vi "Orca Flash Capture Manager.vi"(7 "Calling VI Ref":refnum<vi>) -> ()   [LabVIEW 2016]
uses:
  Orca Flash Capture Manager Controls/Orca Flash Capture Switch Line Scan Modes.ctl
  Orca Flash Capture Manager Controls/Orca Flash Capture Line Scan Settings.ctl
  Orca Flash Capture Manager Controls/Orca Flash Switch Cycles Steps.ctl
  <vilib>/Utility/miscctls.llb/LVPointTypeDef.ctl
  Orca Flash Capture Manager Controls/Orca Flash Capture Notifier Type.ctl
  Orca Flash Capture Manager Controls/Orca Flash Capture Actions.ctl
  <vilib>/vision/Image Controls.llb/IMAQ Image.ctl
  Hardware Configuration/Hardware Configuration Controls/Device Type.ctl
  Orca Flash Capture Manager Controls/Orca Flash Capture Line Scan Filter Settings.ctl
  Hardware Configuration/Hardware Configuration Controls/Device Function.ctl
  Device Library/Cameras/Hamamatsu/Orca Flash/Orca Flash Controls/Orca Flash Actions.ctl
  Device Library/Cameras/Hamamatsu/Orca Flash/Orca Flash Controls/Orca Flash Parameters.ctl
  Device Library/Cameras/Hamamatsu/Orca Flash/Orca Flash Controls/Orca Flash Parameter List.ctl
  Device Library/Cameras/Hamamatsu/Orca Flash/Orca Flash Controls/Orca Flash ROI.ctl
  Orca Flash Capture Manager Controls/Orca Flash Capture Cycle Step Count.ctl
  Device Manager/Common Device Queue/Common Device Controls/Common Device Actions.ctl
  Device Library/SMTP Email Alerts/SMTP Email Alerts Type Defs/SMTP Email Alerts Actions.ctl
  Device Library/DAQmx/AO Single Channel Triggered Ramp/AO SCTR Type Defs/AO SCTR Actions.ctl
  Wide Field Drift Correction/WFDC Controls/WFDC External Sync.ctl
  Wide Field Drift Correction/WFDC Controls/WFDC Cycle Pause.ctl
  Wide Field Drift Correction/WFDC Controls/WFDC Status.ctl
  Device Library/Stages/Stages Controls/Stage Actions.ctl
  Device Library/AOTF and AOM/AOTF Controls/AOTF Actions.ctl
  Device Library/Cameras/Camera Controls/Camera IMAQ Key Info.ctl
  <vilib>/Utility/file.llb/Read Delimited Spreadsheet (DBL).vi
  shell32.dll
panel:
  in  "Main Tab":T1(tab)
  in  "Scan Mode":T2=enum."Cycles Then Steps"
  out "Frame":u32(slide) scale=0.0..20.0
  out "Cycle":sgl(slide) scale=0.0..1.0
  in  "Base Save Path":path
  in  "Capture":bool
  in  "Live Preview":bool
  out "Z Step":sgl(slide) scale=0.0..1.0
  in  "File Name":string="Test Image"
  in  "Preview Exposure Time (s)":dbl=0.1 caption="Frame Rate (Hz)"
  in  "Capture Exposure Time (s)":dbl=0.1 caption="Frame Rate (Hz)"
  in  "No. of Frames":u32=1 min=1
  in  "No. of Cycles":u16=1 min=1
  in  "No. of Z Steps":u16=1 min=1
  in  "Z Step Size (µm)":dbl min=-10.0 max=10.0
  out "Current Cycle":u16
  out "Current Step":u16
  out "Current Frame":u32
  in  "Auto Update Subfolder":bool=TRUE
  in  "Subfolder Name":string="Area"
  in  "Current Filter":i32(ring) items=["Quad Band", "Cy3 / Cy5"]
  in  "Save As Preset":bool
  in  "Line Scan Active":bool
  in  "Number of Lines":u32=8 min=1 max=200 step=1
  in  "Line Scan Mode":T3
  in  "Line Scanning Presets":u16(ring) items=["04 FPS", "08 FPS Clean", "08 FPS", "40 FPS"]
  in  "Line Scan Settings":T4
  in  "Camera Settings":bool
  in  "Quadrants On/Off":bool
  in  "Email Alerts":bool
  in  "Email Address":string
  in  "Quit":bool
  # "Live Preview"
  # "Capture"
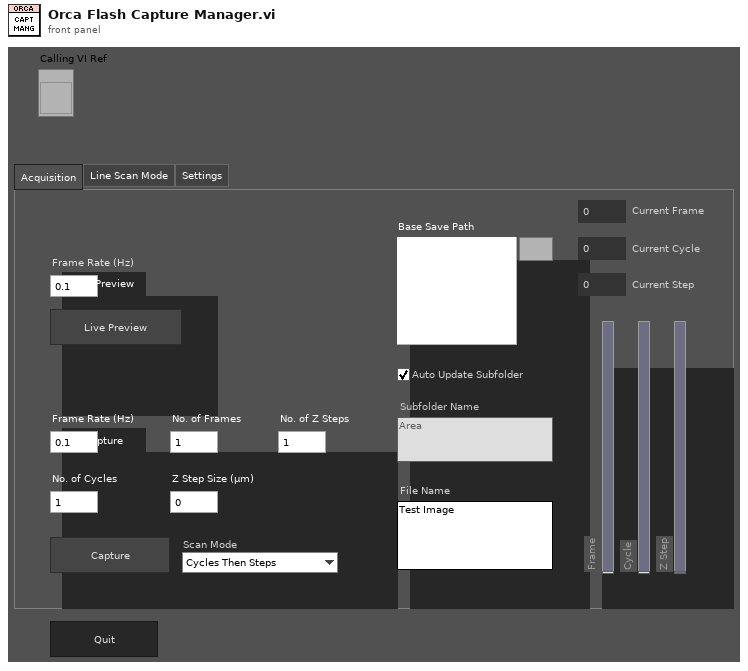
[diagram p1: front panel]
types:
  T1 = enum32{"Acquisition", "Line Scan Mode", "Settings"}
  T2 = typedef "Orca Flash Switch Cycles Steps.ctl" = enum16{"Steps Then Cycles", "Cycles Then Steps"}
  T3 = typedef "Orca Flash Capture Switch Line Scan Modes.ctl" = enum32{"Automatic", "Use Presets", "Manual"}
  T4 = typedef "Orca Flash Capture Line Scan Settings.ctl" = cluster{"Interline Interval":dbl, "Offset (V)":dbl, "Amplitude (V)":dbl, "Samples Per Channel":dbl, "Delay (ms)":dbl}
  T5 = typedef "IMAQ Image.ctl" = refnum<image>
  T6 = cluster{"Image Ref":T5, "Cycle Number":u16, "Camera Running?":bool, "Capture?":bool}
  T7 = typedef "Orca Flash Capture Line Scan Filter Settings.ctl" = cluster{"Filter Name":string, "Offset (V)":dbl}[]
  T8 = enum8{"Enabled", "Disabled", "Disabled and Grayed Out"}
  T9 = typedef "Device Type.ctl" = enum16{"AOTF", "Camera", "Deformable Mirror", "Laser", "Shutter", "Stage", "Waveform", "Email"}
  T10 = typedef "Orca Flash Capture Notifier Type.ctl" = cluster{"Actions":T11, "Running?":bool, "Preview Exposure (s)":dbl, "Capture Exposure (s)":dbl, "Cycles":u16, "Frames":u32, "No. of Z Steps":u16, "Z Step Size (µm)":dbl, "Base Path":path, "Init Z Position (µm)":dbl, "Lasers Lines":string[], "Save Path":path, "Line Scan?":bool, "Line Scan Mode":T3}
  T11 = typedef "Orca Flash Capture Actions.ctl" = enum16{"Idle", "Live Preview", "Capture", "Laser On", "Laser Off", "Open Shutters", "Close Shutters", "Set Exposure Time", "Start Acquisition", "Update SubFolder", "Write Metadata", "Setup", "Camera", "Switch", "Step", "Cycle", "External Cycle Sync", "Abort", "Quit"}
  T12 = enum16{"Always On", "Always Off", "Off While Running"}
  T13 = typedef "LVPointTypeDef.ctl" = cluster{"Horizontal":i16, "Vertical":i16}
  T14 = typedef "Image Type" = u32
  T15 = typedef "Device Function.ctl" = enum16{"Primary", "Secondary", "Overview", "Wide Field Drift Correction", "642 nm Excitation", "560 nm Excitation", "546 nm Excitation", "488 nm Excitation", "405 nm Excitation", "Objective Drift Correction", "4Pi Objective Lock", "Objective XY", "Objective Z", "Sample XY", "Sample Coarse Z", "Sample Z", "4Pi Lower", "4Pi Upper", "Adj Cavity", "Line Scanning", "Alert"}
  T16 = typedef "Orca Flash ROI.ctl" = cluster{"H Offset":i32, "V Offset":i32, "H Width":i32, "V Width":i32}
  T17 = typedef "Orca Flash Parameters.ctl" = cluster{"Value":dbl, "Parameter":T18}
  T18 = typedef "Orca Flash Parameter List.ctl" = u32
  T19 = typedef "Orca Flash Actions.ctl" = enum16{"IDLE", "PREVIEW", "RECORD", "Record Settings", "SETPARAM", "GETPARAM", "SETROI", "GETROI", "PROGRESSIVE MODE", "AREA MODE", "STATUS", "QUIT"}
  T20 = typedef "Orca Flash Capture Cycle Step Count.ctl" = cluster{"Scan Mode":T2, "Current Step":u16, "Current Cycle":u16, "Num of Steps":u16, "Num of Cycles":u16}
  T21 = typedef "WFDC Status.ctl" = enum16{"Idle", "Busy", "DC Active", "Error"}
  T22 = typedef "WFDC External Sync.ctl" = cluster{"Cycle Sync":T23, "Z Offset":dbl, "WFDC Status":T21}
  T23 = typedef "WFDC Cycle Pause.ctl" = enum16{"Pause Requested", "Paused", "Resume Requested", "Resumed"}
  T24 = typedef "SMTP Email Alerts Actions.ctl" = enum16{"Set Recipient", "Send Message", "Quit"}
  T25 = typedef "Stage Actions.ctl" = enum16{"Get Position", "MVR", "MOVE", "HALT", "ONTARGET", "ERROR", "REFERENCE", "INIT", "VELOCITY", "STATUS", "EXIT", "HOME", "ZEROPOS", "NANOPOS", "ANALOG", "QUIT"}
  T26 = typedef "AOTF Actions.ctl" = enum16{"Error Check", "Blank", "Line On/Off", "Set Power", "Status", "Quit"}
  T27 = typedef "AO SCTR Actions.ctl" = enum16{"Stop at Offset", "Update and Run", "Quit"}
  T28 = typedef "Camera IMAQ Key Info.ctl" = cluster{"Frame":u32, "Sensor Height":i32, "Sensor Width":i32, "ROI Height":i32, "ROI Width":i32, "ROI Enable?":bool, "Bit per Pixel":u8}
  T29 = typedef "Common Device Actions.ctl" = enum16{"Open Front Panel", "Close Front Panel", "Quit", "Quit All"}
  T30 = typedef "LVRectTypeDef.ctl" = cluster{"Left":i16, "Top":i16, "Right":i16, "Bottom":i16}
  T31 = typedef "LVBoundsTypeDef.ctl" = cluster{"Width":u32, "Height":u32}
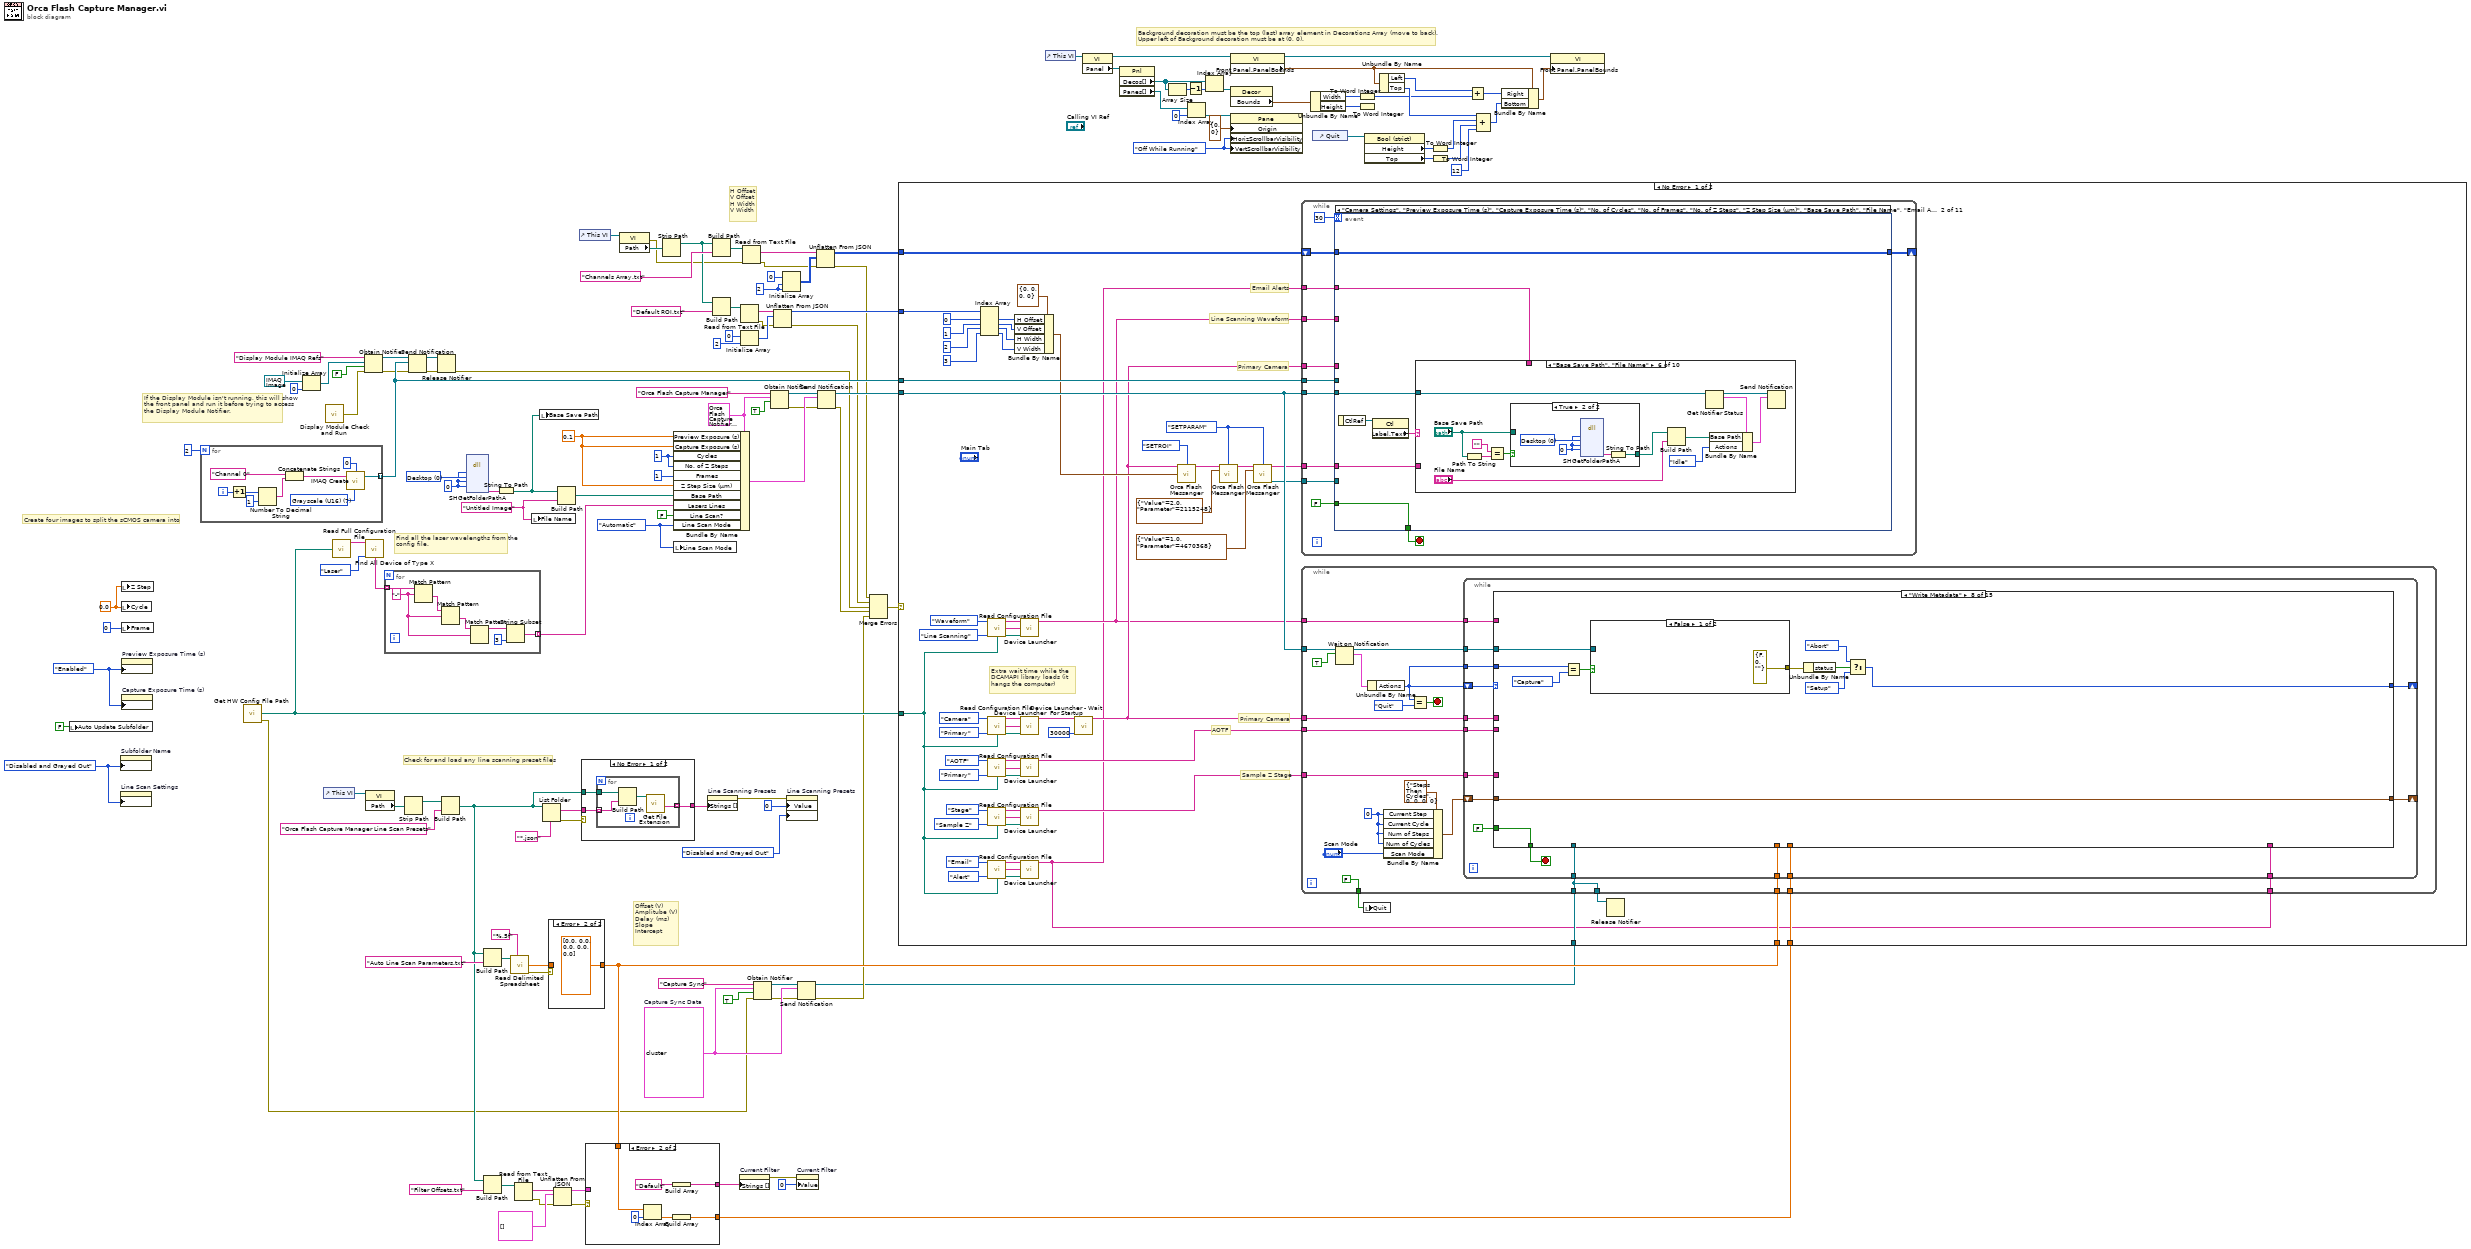
[diagram p0: block diagram]
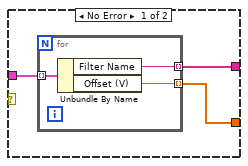
[diagram p2: hidden frame]
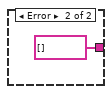
[diagram p4: hidden frame]
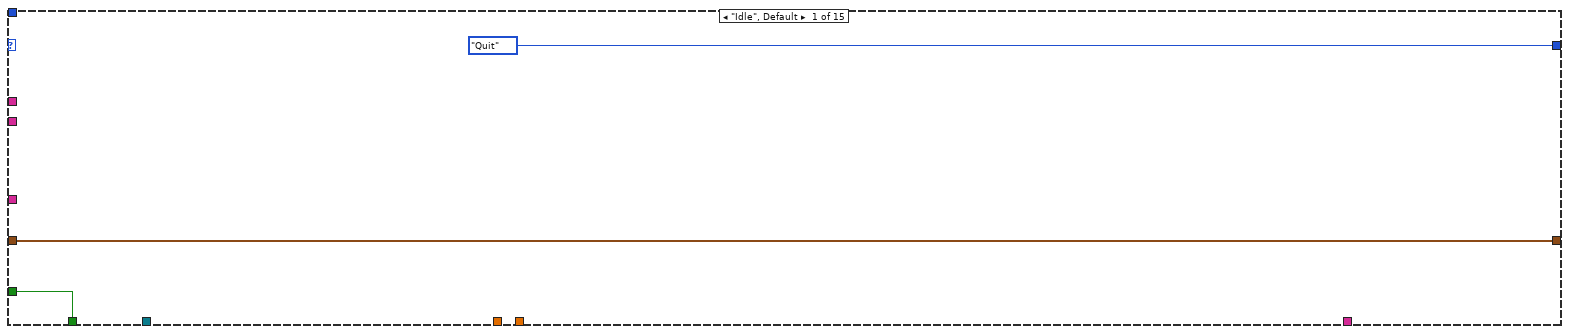
[diagram p5: hidden frame]
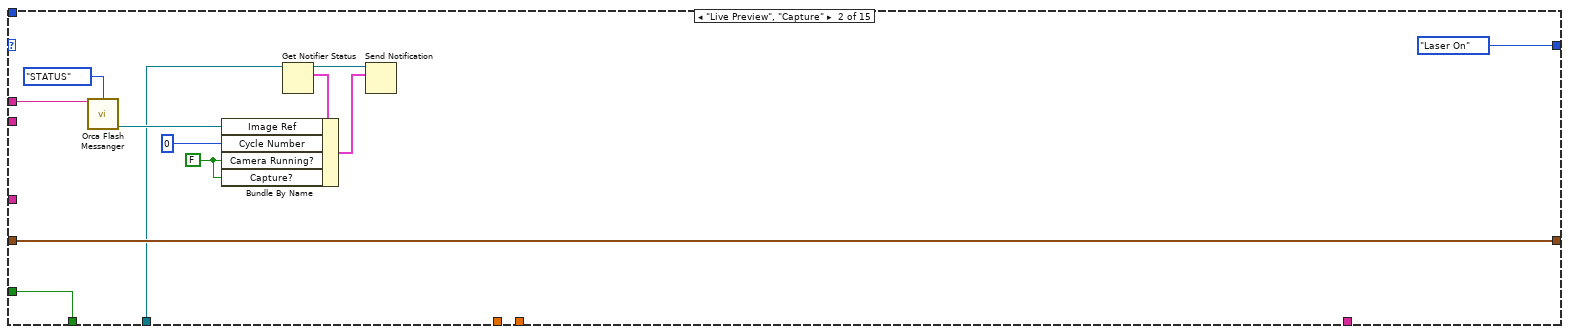
[diagram p6: hidden frame]
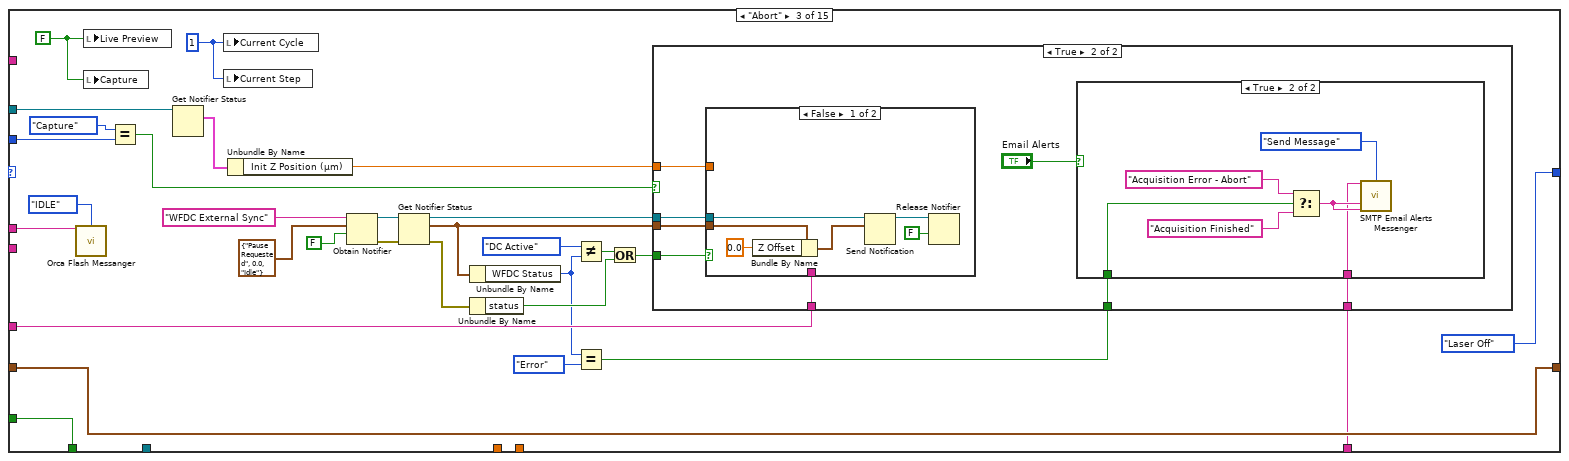
[diagram p7: hidden frame]
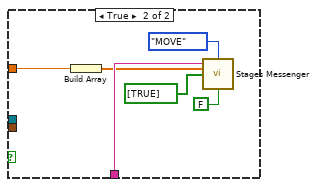
[diagram p10: hidden frame]
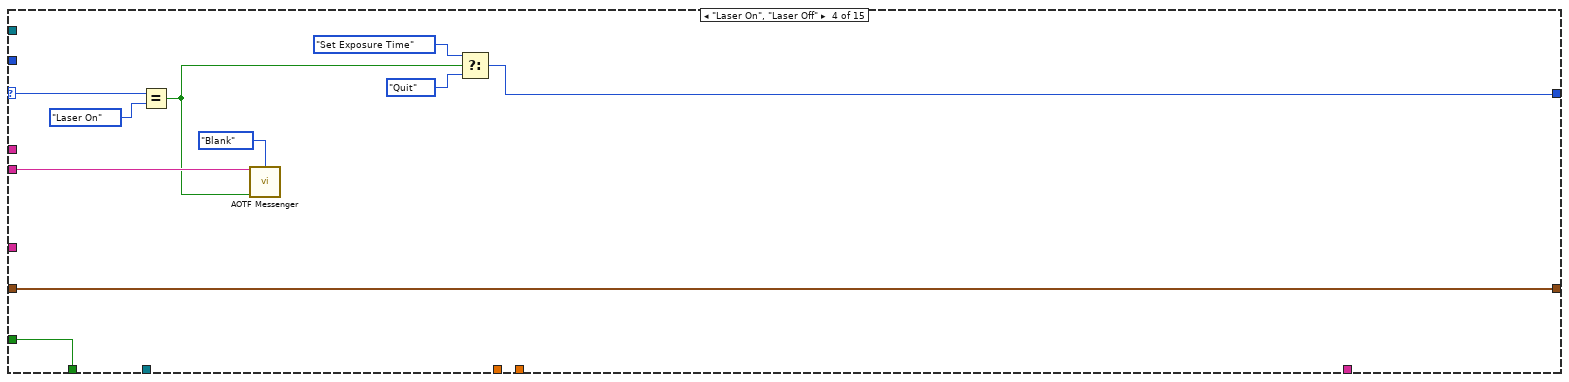
[diagram p11: hidden frame]
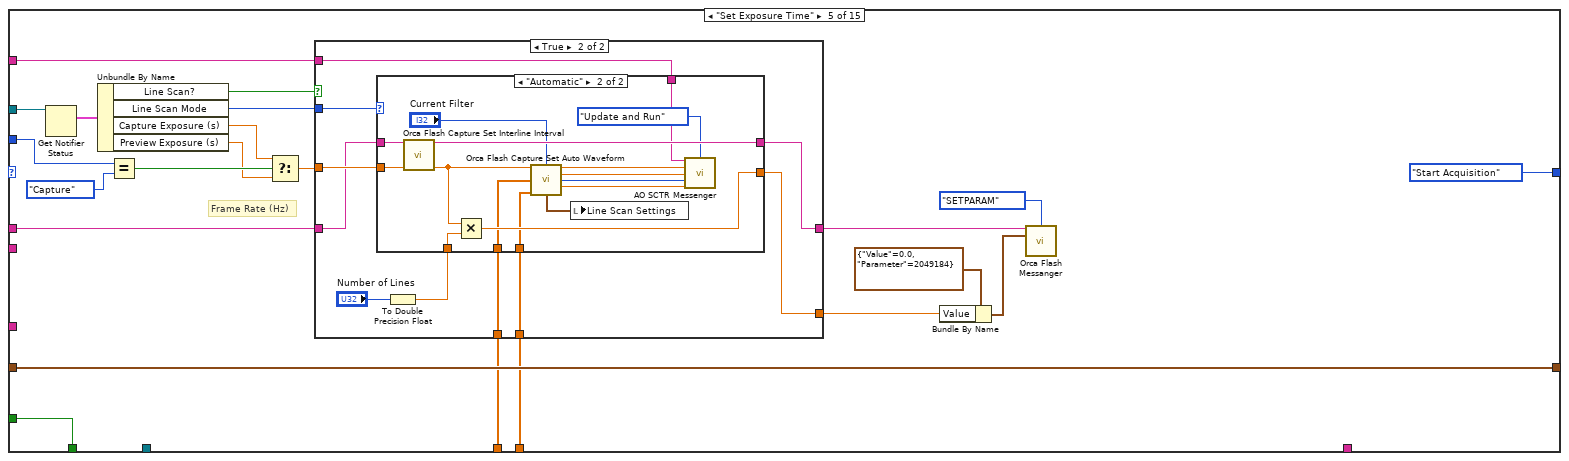
[diagram p12: hidden frame]
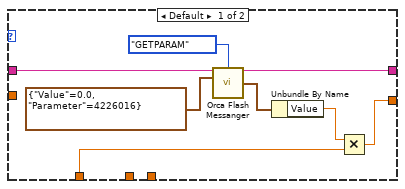
[diagram p14: hidden frame]
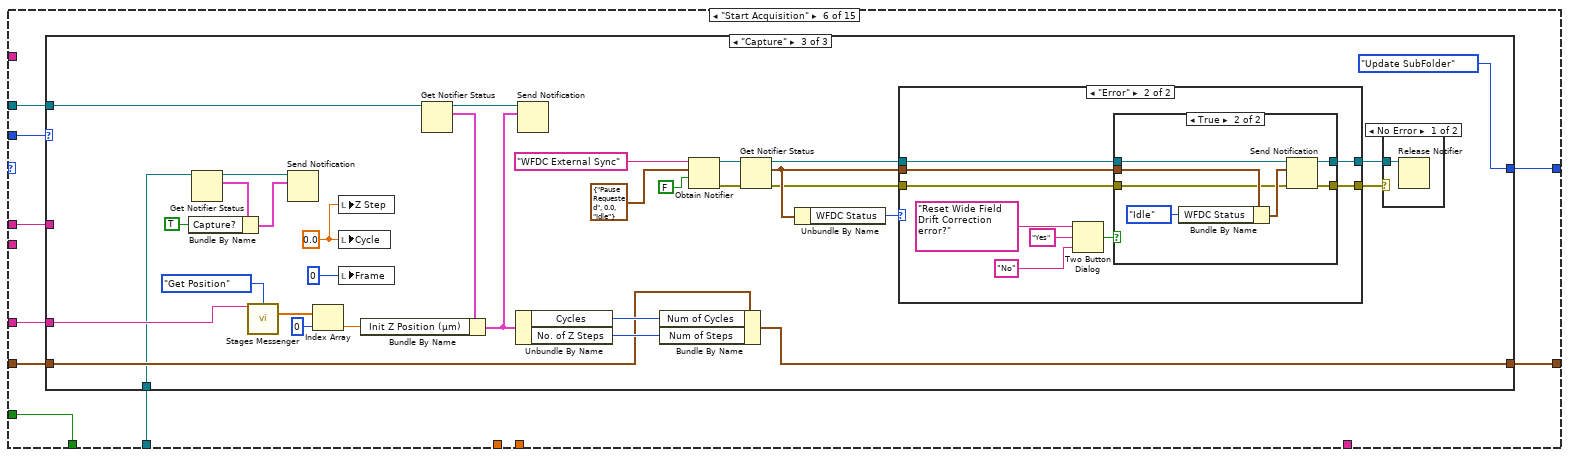
[diagram p15: hidden frame]
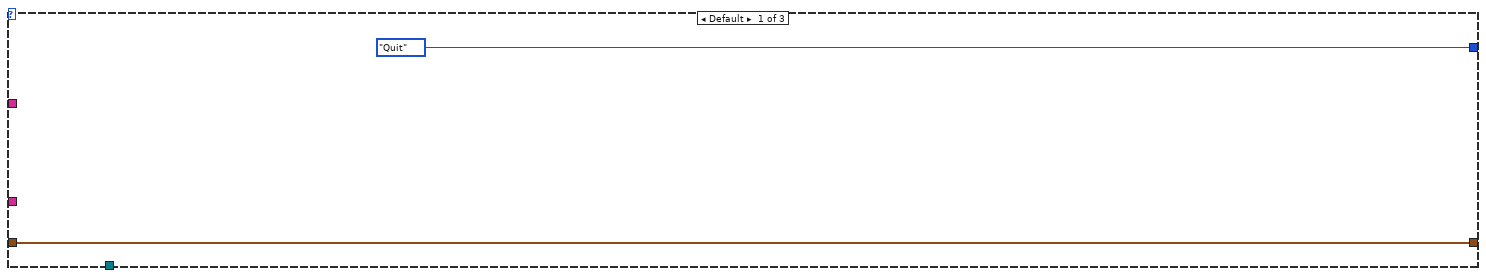
[diagram p16: hidden frame]
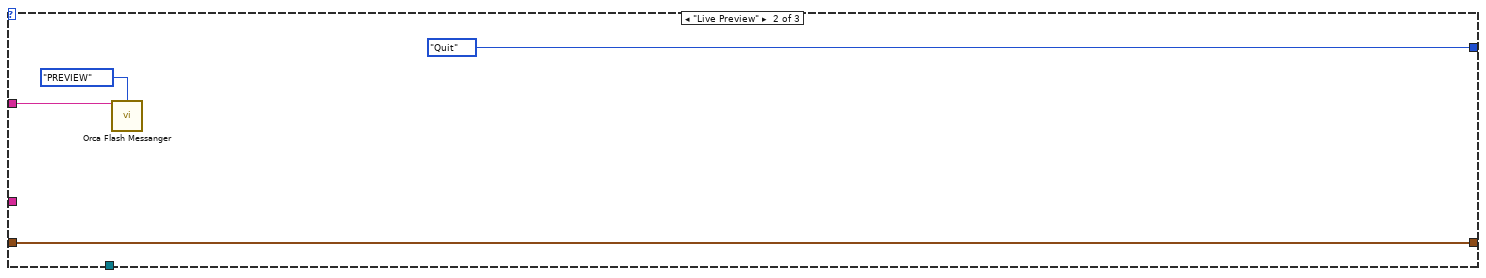
[diagram p17: hidden frame]
diagram:
  w6 = sgl 0.0 ("Cycle")
  w7 = T6 {"Image Ref"=refnum, "Cycle Number"=0, "Camera Running?"=FALSE, "Capture?"=FALSE}  # Capture Sync Data
  w29 = T8."Enabled" ("Disabled")
  w30 = Orca_Flash_Capture_Switch_Line_Scan_Modes."Automatic" ("Line Scan Mode")
  w31 = T8."Disabled and Grayed Out" ("Disabled")
  w79 = 2 ("dimension size")
  w83 = "Untitled Image"
  w86 = 0 items=["Desktop"=0, "Personal Documents"=5, "AppData"=26, "Local AppData"=28, "Common AppData"=35, "Program Files"=38, "Program Files Common"=43, "Common Documents"=46] ("Requested Path")
  w85 = 0 ("HWND")
  w90 = u16 1 ("Cycles")
  w88 = 0.1 ("Preview Exposure (s)")
  w92 = T10 {"Actions"=enum."Live Preview", "Running?"=FALSE, "Preview Exposure (s)"=0.1, "Capture Exposure (s)"=0.1, "Cycles"=1, "Frames"=0, "No. of Z Steps"=0, "Z Step Size (µm)"=0.0, "Base Path"=path "", "Init Z Position (µm)"=0.0, "Lasers Lines"=[], "Save Path"=path "", "Line Scan?"=FALSE, "Line Scan Mode"=enum."Automatic"} ("4Pi Capture Notifier Type")
  w114 = T12."Off While Running" ("Vertical Scrollbar Visibility")
  # "Offset (V)\nAmplitube (V)\nDelay (ms)\nSlope\nIntercept"
  # "Check for and load any line scanning preset files"
  # "Find all the laser wavelengths from the config file."
  # "If the Display Module isn't running, this will show the front panel and run it before trying to access the Display Module Notifier."
  # "H Offset\nV Offset\nH Width\nV Width"
  # "Create four images to split the sCMOS camera into"
  # "Background decoration must be the top (last) array element in Decorations Array (move to back).\nUpper left of Background decoration must be at (0, 0)."
  n1 = local write "Auto Update Subfolder"(FALSE ("Auto Update Subfolder")) -> ()
  n2 = property on="Subfolder Name" class="Str"("DisabledEnum"=w31) -> ()  [unwired: 2 in, 2 out]
  n3 = property on="Line Scan Settings" class="Clust (strict)"("DisabledEnum"=w31) -> ()  [unwired: 2 in, 2 out]
  n4 = local write "Z Step"(w6) -> ()
  n5 = local write "Cycle"(w6) -> ()
  n6 = local write "Frame"(u32 0 ("Frame")) -> ()
  n7 = property on="Preview Exposure Time (s)" class="DigNum (strict)"("DisabledEnum"=w29) -> ()  [unwired: 2 in, 2 out]
  n8 = property on="Capture Exposure Time (s)" class="DigNum (strict)"("DisabledEnum"=w29) -> ()  [unwired: 2 in, 2 out]
  n9 = for {
    N: 2 -> [_]
    tunnel: [w132] -> w96 mode=indexing
    i -> [w140]
    w135 = T14 7 items=["Grayscale (U8)", "Grayscale (I16)", "Grayscale (SGL)", "Complex (CSG)", "RGB (U32)", "HSL (U32)", "RGB (U64)", "Grayscale (U16)"] ("Image Type")
    n10 = Increment(x=w140) -> (x+1=w138:i32)
    n11 = Number To Decimal String(number=w138, width (-)=i16 1) -> (decimal integer string=w136:string)
    n12 = Concatenate Strings("Channel 0" ("name (unnamed)"), w136) -> (w133:string)
    n13 = call "IMAQ Create"("Border Size"=0, "Image Name"=w133, "Image Type"=w135) -> ("New Image"=w132:T5)  [unwired: 2 in, 1 out]
  }
  n14 = call "Get HW Config File Path.vi"() -> ("File Path"=w45:path, "Error"=w4:errorcluster)  [unwired: 14 in]
  n15 = Initialize Array(T5 refnum ("New Image"), 0 ("dimension size")) -> (w51:T5[])
  n16 = control-ref of="This VI"() -> (w42:refnum<vi>)
  n17 = call "Display Module Check and Run.vi"() -> ("Error"=w50:errorcluster)  [unwired: 15 in]
  n18 = call "Read Full Configuration File.vi"("Config File Path"=w45) -> ("Unique Notifier Names"=w47:string[])  [unwired: 11 in, 3 out]
  n19 = Obtain Notifier(name (unnamed)="Display Module IMAQ Refs", notification data type=w51, create if not found? (T)=FALSE, error in (no error)=w50) -> (notifier out=w97:refnum<notifier>, error out=w61:errorcluster)  [unwired: 1 out]
  n20 = call "Find All Device of Type X.vi"("Unique Notifier Names"=w47, "Device Type"=Device_Type."Laser") -> ("All Devices"=w49:string[])  [unwired: 12 in, 1 out]
  n21 = property class="VI"(reference=w42) -> ("Path"=w41:path)  [unwired: 1 in, 2 out]
  n22 = for {
    tunnel: w49 -> [w142] mode=indexing
    tunnel: [w141] -> w46 mode=indexing
    w145 = "-" ("regular expression")
    n23 = Match Pattern(string=w142, regular expression=w145) -> (after substring=w143:string)  [unwired: 1 in, 3 out]
    n24 = Match Pattern(string=w143, regular expression=w145) -> (after substring=w144:string)  [unwired: 1 in, 3 out]
    n25 = Match Pattern(string=w144, regular expression=w145) -> (before substring=w146:string)  [unwired: 1 in, 3 out]
    n26 = String Subset(string=w146, length (rest)=3 ("length (rest)")) -> (substring=w141:string)  [unwired: 1 in]
  }
  n27 = Strip Path(path=w41) -> (stripped path=w40:path)  [unwired: 1 out]
  n28 = Send Notification(notification=w96, notifier=w97, error in (no error)=w61) -> (notifier out=w81:refnum<notifier>, error out=w66:errorcluster)
  n29 = Release Notifier(notifier=w81, error in (no error)=w66) -> (error out=w58:errorcluster)  [unwired: 1 in, 2 out]
  n30 = Build Path(base path=w40, name or relative path="Orca Flash Capture Manager Line Scan Presets") -> (appended path=w23:path)
  n31 = dll-call lib="shell32.dll" fn="SHGetFolderPathA"("HWND"=w85, "nFolder"=w86, "hToken"=w85, "dwFlags"=w85) -> ("pszPath"=w84:string)  [unwired: 9 in, 2 out]
  n32 = Build Path(base path=w23, name or relative path="Auto Line Scan Parameters.txt") -> (appended path=w27:path)
  n33 = Build Path(base path=w23, name or relative path="Filter Offsets.txt") -> (appended path=w21:path)
  n34 = String To Path(string=w84) -> (path=w82:path)
  n35 = call-poly <vilib>:"Read Delimited Spreadsheet.vi"("file path (dialog if empty)"=w27, "format (%.3f)"="%.5f") -> ("first row"=w24:dbl[], "error out"=w25:errorcluster)  [unwired: 8 in, 4 out]
  n36 = Read from Text File(file (use dialog)=w21) -> (text=w20:string, error out=w18:errorcluster)  [unwired: 3 in, 2 out]
  n37 = local write "File Name"(w83) -> ()
  n38 = local write "Base Save Path"(w82) -> ()
  n39 = List Folder(path=w23, pattern="*.json") -> (filenames=w37:string[], error out=w36:errorcluster)  [unwired: 2 in, 2 out]
  n40 = case shown="Error" w25 {
    tunnel: w24 -> [w148 _]
    tunnel: [w148 dbl[] [0.0, 0.0, 0.0, 0.0, 0.0] ("first row")] -> w15
    frame No Error {
    }
    frame Error {
    }
  }
  n41 = Unflatten From JSON(JSON string=w20, type and defaults=T7 [] ("Line Scan Filter Parameters"), error in (no error)=w18) -> (value=w17:T7, error out=w16:errorcluster)  [unwired: 4 in]
  n42 = Build Path(base path=w82, name or relative path=w83) -> (appended path=w87:path)
  n43 = control-ref of="This VI"() -> (w95:refnum<vi>)
  n44 = case shown="No Error" w36 {
    tunnel: w37 -> [w152 _]
    tunnel: w23 -> [w151 _]
    tunnel: [w150 string[] []] -> w35
    frame No Error {
      n45 = for {
        tunnel: w152 -> [w155] mode=indexing
        tunnel: w151 -> [w156]
        tunnel: [w153] -> w150 mode=indexing
        n46 = Build Path(base path=w156, name or relative path=w155) -> (appended path=w154:path)
        n47 = call <vilib>:"Get File Extension.vi"("file"=w154) -> ("filename without extension"=w153:string)  [unwired: 6 in, 4 out]
      }
    }
    frame Error {
    }
  }
  n48 = case shown="Error" w16 {
    tunnel: w17 -> [w160 _]
    tunnel: w15 -> [_ w168]
    tunnel: [w159 w165] -> w14
    tunnel: [w158 w164] -> w11
    frame No Error {
      n49 = for {
        tunnel: w160 -> [w163] mode=indexing
        tunnel: [w162] -> w159 mode=indexing
        tunnel: [w161] -> w158 mode=indexing
        n50 = Unbundle By Name(w163) -> ("Filter Name"=w162:string, "Offset (V)"=w161:dbl)
      }
    }
    frame Error {
      n51 = Index Array(array=w168, index=0) -> (element=w166:dbl)
      n52 = Build Array("Default") -> (w165:string[])
      n53 = Build Array(w166) -> (w164:dbl[])
    }
  }
  n54 = property class="VI"(reference=w95) -> (error out=w63:errorcluster, "Path"=w94:path)  [unwired: 1 in, 1 out]
  n55 = Strip Path(path=w94) -> (stripped path=w74:path)  [unwired: 1 out]
  n56 = Bundle By Name(cluster=w92, "Preview Exposure (s)"=w88, "Capture Exposure (s)"=w88, "Cycles"=w90, "No. of Z Steps"=w90, "Frames"=u32 1, "Z Step Size (µm)"=w88, "Base Path"=w87, "Lasers Lines"=w46, "Line Scan?"=FALSE, "Line Scan Mode"=w30) -> (w91:T10)
  n57 = local write "Line Scan Mode"(w30) -> ()
  n58 = property on="Line Scanning Presets" class="Ring (strict)"("Strings []"=w35) -> (error out=w34:errorcluster)  [unwired: 2 in, 1 out]
  n59 = Build Path(base path=w74, name or relative path="Channels Array.txt") -> (appended path=w77:path)
  n60 = Build Path(base path=w74, name or relative path="Default ROI.txt") -> (appended path=w72:path)
  n61 = property on="Current Filter" class="Ring (strict)"("Strings []"=w14) -> (error out=w13:errorcluster)  [unwired: 2 in, 1 out]
  n62 = Read from Text File(file (use dialog)=w72) -> (text=w71:string, error out=w64:errorcluster)  [unwired: 3 in, 2 out]
  n63 = Initialize Array(0 ("element"), 2 ("dimension size")) -> (w68:i32[])
  n64 = Read from Text File(file (use dialog)=w77, error in=w63) -> (text=w76:string, error out=w62:errorcluster)  [unwired: 2 in, 2 out]
  n65 = Obtain Notifier(name (unnamed)="Capture Sync", notification data type=w7, create if not found? (T)=TRUE, error in (no error)=w4) -> (notifier out=w8:refnum<notifier>, error out=w3:errorcluster)  [unwired: 1 out]
  n66 = Obtain Notifier(name (unnamed)="Orca Flash Capture Manager", notification data type=w92, create if not found? (T)=TRUE) -> (notifier out=w100:refnum<notifier>, error out=w65:errorcluster)  [unwired: 1 in, 1 out]
  n67 = Unflatten From JSON(JSON string=w71, type and defaults=w68, error in (no error)=w64) -> (value=w67:i32[], error out=w57:errorcluster)  [unwired: 4 in]
  n68 = Initialize Array(0 ("element"), w79, w79) -> (w78:i32[][])
  n69 = property on="Line Scanning Presets" class="Ring (strict)"(error in=w34, "Value"=u16 0, "DisabledEnum"=T8."Disabled and Grayed Out" ("Disabled")) -> ()  [unwired: 1 in, 2 out]
  n70 = property on="Current Filter" class="Ring (strict)"(error in=w13, "Value"=0) -> ()  [unwired: 1 in, 2 out]
  n71 = Send Notification(notification=w7, notifier=w8, error in (no error)=w3) -> (notifier out=w1:refnum<notifier>, error out=w2:errorcluster)
  n72 = Unflatten From JSON(JSON string=w76, type and defaults=w78, error in (no error)=w62) -> (value=w75:i32[][], error out=w56:errorcluster)  [unwired: 4 in]
  n73 = Send Notification(notification=w91, notifier=w100, error in (no error)=w65) -> (notifier out=w99:refnum<notifier>, error out=w59:errorcluster)
  n74 = Merge Errors(w56, w57, w58, w59, w2) -> (w60:errorcluster)
  n75 = case shown="No Error" w60 {
    tunnel: w45 -> [w171 _]
    tunnel: w99 -> [w219 w1101]
    tunnel: w96 -> [w209 w1099]
    tunnel: w75 -> [w208 _]
    tunnel: w67 -> [w199 _]
    tunnel: w15 -> [w180 _]
    tunnel: w11 -> [w179 _]
    tunnel: w1 -> [w178 _]
    frame No Error {
      w204 = Orca_Flash_Actions."SETPARAM" ("Camera Actions")
      # "Email Alerts"
      # "Line Scanning Waveform"
      # "Primary Camera"
      # "Extra wait time while the DCAMAPI library loads (it hangs the computer)"
      # "Sample Z Stage"
      # "AOTF"
      # "Primary Camera"
      n76 = Index Array(array=w199, index #1=0 ("index"), index #2=1 ("index"), index #3=2 ("index"), index #4=3 ("index")) -> (element #1=w194:i32, element #2=w191:i32, element #3=w192:i32, element #4=w193:i32)
      n77 = call "Read Configuration File.vi"("Device Type"=Device_Type."Waveform", "Device Function"=Device_Function."Line Scanning", "Config File Path"=w171) -> ("Unique Notifier Name"=w184:string, "Device Ports/IDs/Channels"=w185:string[], "Device Engine Path"=w182:path)  [unwired: 9 in, 1 out]
      n78 = call "Read Configuration File.vi"("Device Type"=Device_Type."Camera", "Device Function"=Device_Function."Primary", "Config File Path"=w171) -> ("Unique Notifier Name"=w229:string, "Device Ports/IDs/Channels"=w228:string[], "Device Engine Path"=w227:path)  [unwired: 9 in, 1 out]
      n79 = call "Read Configuration File.vi"("Device Type"=Device_Type."AOTF", "Device Function"=Device_Function."Primary", "Config File Path"=w171) -> ("Unique Notifier Name"=w220:string, "Device Ports/IDs/Channels"=w221:string[], "Device Engine Path"=w222:path)  [unwired: 9 in, 1 out]
      n80 = call "Read Configuration File.vi"("Device Type"=Device_Type."Stage", "Device Function"=Device_Function."Sample Z", "Config File Path"=w171) -> ("Unique Notifier Name"=w216:string, "Device Ports/IDs/Channels"=w214:string[], "Device Engine Path"=w213:path)  [unwired: 9 in, 1 out]
      n81 = call "Read Configuration File.vi"("Device Type"=Device_Type."Email", "Device Function"=Device_Function."Alert", "Config File Path"=w171) -> ("Unique Notifier Name"=w174:string, "Device Ports/IDs/Channels"=w173:string[], "Device Engine Path"=w176:path)  [unwired: 9 in, 1 out]
      n82 = Bundle By Name(cluster=T16 {"H Offset"=0, "V Offset"=0, "H Width"=0, "V Width"=0} ("Orca Flash ROI"), "H Offset"=w194, "V Offset"=w191, "H Width"=w192, "V Width"=w193) -> (w190:T16)
      n83 = call "Device Launcher.vi"("Notifier Name"=w184, "Device Ports/IDs/Channels"=w185, "Device Engine Path"=w182) -> ("Notifier Name"=w181:string)  [unwired: 11 in, 1 out]
      n84 = call "Device Launcher.vi"("Notifier Name"=w229, "Device Ports/IDs/Channels"=w228, "Device Engine Path"=w227) -> ("Notifier Name"=w188:string)  [unwired: 11 in, 1 out]
      n85 = call "Device Launcher.vi"("Notifier Name"=w220, "Device Ports/IDs/Channels"=w221, "Device Engine Path"=w222) -> ("Notifier Name"=w218:string)  [unwired: 11 in, 1 out]
      n86 = call "Device Launcher.vi"("Notifier Name"=w216, "Device Ports/IDs/Channels"=w214, "Device Engine Path"=w213) -> ("Notifier Name"=w211:string)  [unwired: 11 in, 1 out]
      n87 = call "Device Launcher.vi"("Notifier Name"=w174, "Device Ports/IDs/Channels"=w173, "Device Engine Path"=w176) -> ("Notifier Name"=w170:string)  [unwired: 11 in, 1 out]
      n88 = call "Device Launcher - Wait For Startup.vi"("Notifier Name"=w188, "Wait Time (ms)"=30000) -> ("Notifier Name (Dup)"=w187:string)  [unwired: 12 in, 1 out]
      n89 = call "Orca Flash Messanger.vi"("Notifier Name"=w187, "Camera Actions"=Orca_Flash_Actions."SETROI", "sCMOS ROI"=w190) -> ("Notifier Name Dup"=w207:string)  [unwired: 8 in, 4 out]
      n90 = call "Orca Flash Messanger.vi"("Notifier Name"=w207, "Camera Actions"=w204, "sCMOS Parameter"=T17 {"Value"=2.0, "Parameter"=2115248}) -> ("Notifier Name Dup"=w206:string)  [unwired: 8 in, 4 out]
      n91 = call "Orca Flash Messanger.vi"("Notifier Name"=w206, "Camera Actions"=w204, "sCMOS Parameter"=T17 {"Value"=1.0, "Parameter"=4670368}) -> ("Notifier Name Dup"=w205:string, "Image Ref"=w201:T5)  [unwired: 8 in, 3 out]
      n92 = while {
        tunnel: w219 -> [w776]
        tunnel: w205 -> [w775]
        tunnel: w201 -> [w773]
        tunnel: w209 -> [w772]
        shift-right: [w770] -> _
        shift-left: w208 -> [w771]
        tunnel: w187 -> [w769]
        tunnel: w181 -> [w768]
        tunnel: w170 -> [w767]
        stop <- w778 stop-if-true
        n93 = event shown="[1] \"Camera Settings\", \"Preview Exposure Time (s)\", \"Capture Exposure Time (s)\", \"No. of Cycles\", \"No. of Frames\", \"No. of Z Steps\", \"Z Step Size (µm)\", \"Base Save Path\", \"File Name\", \"Email Address\": Value Change" {
          selector: _ -> [_ _ _ _ _ _ _ _ _ _ _]
          dyn-events: _ -> [_ _ _ _ _ _ _ _ _ _ _]
          timeout: 30 -> [_ _ _ _ _ _ _ _ _ _ _]
          tunnel: [w783 w802 w878 w899 w955 w980 w1002 w1018 w1042 w1066 w1097] -> w778
          tunnel: FALSE -> [w783 w802 w878 w899 w955 w980 w1002 w1018 w1042 w1066 _]
          tunnel: w776 -> [_ w799 w875 _ _ w974 w1000 _ w1040 _ w1096]
          tunnel: w775 -> [_ w798 _ _ _ _ _ _ _ _ _]
          tunnel: w773 -> [w781 _ _ w883 _ _ _ _ _ _ _]
          tunnel: w772 -> [w782 _ _ w889 _ _ _ _ _ _ w1084]
          tunnel: w771 -> [w780 w797 w867 w882 w950 w957 w1001 w1019 w1041 w1058 w1083]
          tunnel: [w780 w797 w867 w881 w950 w957 w1001 w1019 w1041 w1058 w1083] -> w770
          tunnel: w769 -> [_ _ _ _ _ w968 _ _ w1026 _ _]
          tunnel: w768 -> [_ _ _ _ _ w958 _ _ w1034 _ _]
          tunnel: w767 -> [_ w796 _ _ _ _ _ _ _ _ _]
          event Timeout {
            # "Convert to array and then crop. If you\nextract or mask image the destination\nimage custom data keys are overwritten."
            n94 = event-data() -> ()  [unwired: 1 in, 1 out]
            n95 = call "IMAQ ImageToArray"("Image"=w781) -> ("Image Pixels (U16)"=w779:u16[][])  [unwired: 3 in, 4 out]
            n96 = for {
              tunnel: w782 -> [w794] mode=indexing
              tunnel: w779 -> [w795]
              tunnel: w780 -> [w792] mode=indexing
              n97 = Index Array(array=w792, index #1=0 ("index"), index #2=2 ("index"), index #3=1 ("index"), index #4=3 ("index")) -> (element #1=w790:i32, element #2=w789:i32, element #3=w785:i32, element #4=w784:i32)
              n98 = Array Subset(array=w795, index (row)=w790, length (row)=w789, index (col)=w785, length (col)=w784) -> (w793:u16[][])
              n99 = call "IMAQ ArrayToImage"("Image Pixels (U16)"=w793, "Image"=w794) -> ()  [unwired: 8 in, 2 out]
            }
          }
          event "Camera Settings", "Preview Exposure Time (s)", "Capture Exposure Time (s)", "No. of Cycles", "No. of Frames", "No. of Z Steps", "Z Step Size (µm)", "Base Save Path", "File Name", "Email Address": Value Change {
            n100 = event-data() -> ("CtlRef"=w801:refnum<vi>)  [unwired: 1 in]
            n101 = property class="Ctl"(reference=w801) -> ("Label.Text"=w800:string)  [unwired: 1 in, 2 out]
            n102 = case shown="\"Base Save Path\", \"File Name\"" w800 {
              tunnel: w799 -> [_ w806 w814 w820 w826 w838 _ w854 w863 _]
              tunnel: w798 -> [_ _ _ _ _ _ w846 _ _ _]
              tunnel: w796 -> [_ _ _ _ _ _ _ _ _ w864]
              frame Default {
              }
              frame "No. of Cycles" {
                n103 = Get Notifier Status(notifier=w806) -> (notifier out=w805:refnum<notifier>, current notification=w807:T10)  [unwired: 1 in, 3 out]
                n104 = Bundle By Name(cluster=w807, "Cycles"="No. of Cycles", "Actions"=Orca_Flash_Capture_Actions."Idle") -> (w808:T10)
                n105 = Send Notification(notification=w808, notifier=w805) -> ()  [unwired: 1 in, 2 out]
              }
              frame "No. of Frames" {
                n106 = To Double Precision Float(number="No. of Frames") -> (double precision float=w810:dbl)
                n107 = property on="Frame" class="Slide (strict)"("Scale.Maximum"=w810, "Scale.Minimum"=0.0 ("Scale.Range:Minimum")) -> ()  [unwired: 2 in, 2 out]
                n108 = Get Notifier Status(notifier=w814) -> (notifier out=w813:refnum<notifier>, current notification=w815:T10)  [unwired: 1 in, 3 out]
                n109 = Bundle By Name(cluster=w815, "Frames"="No. of Frames", "Actions"=Orca_Flash_Capture_Actions."Idle") -> (w816:T10)
                n110 = Send Notification(notification=w816, notifier=w813) -> ()  [unwired: 1 in, 2 out]
              }
              frame "No. of Z Steps" {
                n111 = Get Notifier Status(notifier=w820) -> (notifier out=w819:refnum<notifier>, current notification=w821:T10)  [unwired: 1 in, 3 out]
                n112 = Bundle By Name(cluster=w821, "No. of Z Steps"="No. of Z Steps", "Actions"=Orca_Flash_Capture_Actions."Idle") -> (w822:T10)
                n113 = Send Notification(notification=w822, notifier=w819) -> ()  [unwired: 1 in, 2 out]
              }
              frame "Z Step Size (µm)" {
                n114 = Get Notifier Status(notifier=w826) -> (notifier out=w825:refnum<notifier>, current notification=w827:T10)  [unwired: 1 in, 3 out]
                n115 = Bundle By Name(cluster=w827, "Z Step Size (µm)"="Z Step Size (µm)", "Actions"=Orca_Flash_Capture_Actions."Idle") -> (w828:T10)
                n116 = Send Notification(notification=w828, notifier=w825) -> ()  [unwired: 1 in, 2 out]
              }
              frame "Base Save Path", "File Name" {
                n117 = Path To String(path="Base Save Path") -> (string=w833:string)
                n118 = Equal?(x="", y=w833) -> (x = y?=w831:bool)
                n119 = case shown="True" w831 {
                  tunnel: [w841 w842] -> w830
                  tunnel: "Base Save Path" -> [w841 _]
                  frame False {
                  }
                  frame True {
                    w845 = 0 items=["Desktop"=0, "Personal Documents"=5, "AppData"=26, "Local AppData"=28, "Common AppData"=35, "Program Files"=38, "Program Files Common"=43, "Common Documents"=46] ("Requested Path")
                    w844 = 0 ("HWND")
                    n120 = dll-call lib="shell32.dll" fn="SHGetFolderPathA"("HWND"=w844, "nFolder"=w845, "hToken"=w844, "dwFlags"=w844) -> ("pszPath"=w843:string)  [unwired: 9 in, 2 out]
                    n121 = String To Path(string=w843) -> (path=w842:path)
                  }
                }
                n122 = Build Path(base path=w830, name or relative path="File Name") -> (appended path=w834:path)
                n123 = Get Notifier Status(notifier=w838) -> (notifier out=w837:refnum<notifier>, current notification=w839:T10)  [unwired: 1 in, 3 out]
                n124 = Bundle By Name(cluster=w839, "Base Path"=w834, "Actions"=Orca_Flash_Capture_Actions."Idle") -> (w840:T10)
                n125 = Send Notification(notification=w840, notifier=w837) -> ()  [unwired: 1 in, 2 out]
              }
              frame "Camera Settings" {
                n126 = Select(t=Common_Device_Actions."Open Front Panel" ("Common Actions"), s="Camera Settings", f=Common_Device_Actions."Close Front Panel" ("Common Actions")) -> (s? t:f=w850:T29)
                n127 = call "Common Device Queue Messenger.vi"("Common Action"=w850, "Notifier Name"=w846) -> ()  [unwired: 13 in, 1 out]
              }
              frame "Preview Exposure Time (s)" {
                # "Add in a preview stop\nand restart here"
                n128 = Get Notifier Status(notifier=w854) -> (notifier out=w857:refnum<notifier>, current notification=w856:T10)  [unwired: 1 in, 3 out]
                n129 = Bundle By Name(cluster=w856, "Preview Exposure (s)"="Preview Exposure Time (s)", "Running?"=FALSE ("Abort"), "Actions"=Orca_Flash_Capture_Actions."Idle") -> (w855:T10)
                n130 = Send Notification(notification=w855, notifier=w857) -> ()  [unwired: 1 in, 2 out]
              }
              frame "Capture Exposure Time (s)" {
                n131 = Get Notifier Status(notifier=w863) -> (notifier out=w862:refnum<notifier>, current notification=w861:T10)  [unwired: 1 in, 3 out]
                n132 = Bundle By Name(cluster=w861, "Capture Exposure (s)"="Capture Exposure Time (s)", "Actions"=Orca_Flash_Capture_Actions."Idle") -> (w860:T10)
                n133 = Send Notification(notification=w860, notifier=w862) -> ()  [unwired: 1 in, 2 out]
              }
              frame "Email Address" {
                n134 = call "SMTP Email Alerts Messenger.vi"("Notifier Name"=w864, "Actions"=SMTP_Email_Alerts_Actions."Set Recipient", "Recipient"="Email Address") -> ()  [unwired: 13 in]
              }
            }
          }
          event "Live Preview", "Capture": Value Change {
            n135 = event-data() -> ("CtlRef"=w870:refnum<vi>, "NewVal"=w873:bool)  [unwired: 1 in]
            n136 = property class="Bool (strict)"(reference=w870) -> ("Label.Text"=w869:string)  [unwired: 1 in, 2 out]
            n137 = case shown="\"Live Preview\", Default" w869 {
              tunnel: [Orca_Flash_Capture_Actions."Capture" ("y") Orca_Flash_Capture_Actions."Live Preview" ("y")] -> w868
              frame "Capture" {
              }
              frame "Live Preview", Default {
              }
            }
            n138 = Select(t=w868, s=w873, f=Orca_Flash_Capture_Actions."Abort" ("y")) -> (s? t:f=w872:T11)
            n139 = Get Notifier Status(notifier=w875) -> (notifier out=w876:refnum<notifier>, current notification=w874:T10)  [unwired: 1 in, 3 out]
            n140 = Bundle By Name(cluster=w874, "Actions"=w872, "Running?"=w873) -> (w871:T10)
            n141 = Send Notification(notification=w871, notifier=w876) -> ()  [unwired: 1 in, 2 out]
          }
          event "Quadrants On/Off": Value Change {
            n142 = event-data() -> ("NewVal"=w895:bool)  [unwired: 1 in]
            n143 = Obtain Notifier(name (unnamed)="Display Module IMAQ Refs", notification data type=T5[] [], create if not found? (T)=FALSE) -> (notifier out=w888:refnum<notifier>, error out=w887:errorcluster)  [unwired: 1 in, 1 out]
            n144 = Get Notifier Status(notifier=w888, error in (no error)=w887) -> (notifier out=w886:refnum<notifier>, current notification=w884:T5[], error out=w885:errorcluster)  [unwired: 2 out]
            n145 = case shown="True" w895 {
              tunnel: w886 -> [w921 w936]
              tunnel: w885 -> [w920 w935]
              tunnel: [w917 w931] -> w891
              tunnel: [w921 w936] -> w892
              tunnel: [w920 w935] -> w890
              tunnel: w889 -> [w912 w934]
              tunnel: w884 -> [w919 w933]
              tunnel: w883 -> [w913 w930]
              tunnel: w882 -> [_ w929]
              tunnel: [w900 w929] -> w881
              frame False {
                w911 = 2 ("dimension size")
                n146 = control-ref of="This VI"() -> (w901:refnum<vi>)
                n147 = Equal?(x=w919, y=w913) -> (x = y?=w916:bool[])
                n148 = property class="VI"(reference=w901) -> (error out=w909:errorcluster, "Path"=w902:path)  [unwired: 1 in, 1 out]
                n149 = for {
                  tunnel: w916 -> [w928] mode=indexing
                  tunnel: [w927] -> w914
                  i -> [w927]
                  stop <- w928 stop-if-true
                }
                n150 = Or Array Elements(Boolean array=w916) -> (logical OR=w915:bool)
                n151 = Strip Path(path=w902) -> (stripped path=w908:path)  [unwired: 1 out]
                n152 = case shown="True" w915 {
                  tunnel: w914 -> [_ w925]
                  tunnel: w919 -> [w922 w924]
                  tunnel: [w922 w923] -> w918
                  frame False {
                  }
                  frame True {
                    n153 = Delete From Array(array=w924, length=1, index=w925) -> (array with subset deleted=w923:T5[])  [unwired: 1 out]
                  }
                }
                n154 = Build Path(base path=w908, name or relative path="Channels Array.txt") -> (appended path=w906:path)
                n155 = Read from Text File(file (use dialog)=w906, error in=w909) -> (text=w907:string, error out=w910:errorcluster)  [unwired: 2 in, 2 out]
                n156 = Initialize Array(0 ("element"), w911, w911) -> (w905:i32[][])
                n157 = Build Array (concatenate)(w918, w912) -> (w917:T5[])
                n158 = Unflatten From JSON(JSON string=w907, type and defaults=w905, error in (no error)=w910) -> (value=w900:i32[][])  [unwired: 4 in, 1 out]
              }
              frame True {
                n159 = for {
                  tunnel: w934 -> [w939] mode=indexing
                  shift-right: [w937] -> w932
                  shift-left: w933 -> [w938]
                  n160 = Equal?(x=w938, y=w939) -> (x = y?=w942:bool[])
                  n161 = for {
                    tunnel: w942 -> [w949] mode=indexing
                    tunnel: [w948] -> w940
                    i -> [w948]
                    stop <- w949 stop-if-true
                  }
                  n162 = Or Array Elements(Boolean array=w942) -> (logical OR=w941:bool)
                  n163 = case shown="True" w941 {
                    tunnel: w940 -> [_ w946]
                    tunnel: w938 -> [w943 w945]
                    tunnel: [w943 w944] -> w937
                    frame False {
                    }
                    frame True {
                      n164 = Delete From Array(array=w945, length=1, index=w946) -> (array with subset deleted=w944:T5[])  [unwired: 1 out]
                    }
                  }
                }
                n165 = Build Array (concatenate)(w932, w930) -> (w931:T5[])
              }
            }
            n166 = Send Notification(notification=w891, notifier=w892, error in (no error)=w890) -> (notifier out=w894:refnum<notifier>, error out=w893:errorcluster)
            n167 = Release Notifier(notifier=w894, error in (no error)=w893) -> ()  [unwired: 1 in, 3 out]
          }
          event "Auto Update Subfolder": Value Change {
            n168 = event-data() -> ("NewVal"=w954:bool)  [unwired: 1 in]
            n169 = Select(t=T8."Enabled" ("Disabled"), s=w954, f=T8."Disabled and Grayed Out") -> (s? t:f=w951:T8)
            n170 = property on="Subfolder Name" class="Str"("DisabledEnum"=w951) -> ()  [unwired: 2 in, 2 out]
          }
          event "Line Scan Active": Value Change {
            n171 = event-data() -> ("NewVal"=w956:bool)  [unwired: 1 in]
            n172 = Select(t="Frame Rate (Hz)", s=w956, f="Exposure Time (s)") -> (s? t:f=w977:string)
            n173 = Select(t=4.0, s=w956, f=0.1) -> (s? t:f=w970:dbl)
            n174 = Select(t=-1.0 ("f"), s=w956, f=0.0) -> (s? t:f=w961:dbl)
            n175 = Select(t=AO_SCTR_Actions."Update and Run" ("Actions"), s=w956, f=AO_SCTR_Actions."Stop at Offset" ("Actions")) -> (s? t:f=w962:T27)
            n176 = property on="Capture Exposure Time (s)" class="DigNum (strict)"("Caption.Text"=w977, "Value"=w970) -> ()  [unwired: 2 in, 2 out]
            n177 = property on="Preview Exposure Time (s)" class="DigNum (strict)"("Caption.Text"=w977, "Value"=w970) -> ()  [unwired: 2 in, 2 out]
            n178 = call "AO SCTR Messenger.vi"("Notifier Name"=w958, "Actions"=w962, "Offset (V)"=w961) -> ()  [unwired: 12 in, 1 out]
            n179 = case shown="False" w956 {
              frame False {
                w981 = T8."Enabled" ("Disabled")
                n180 = property on="Preview Exposure Time (s)" class="DigNum (strict)"("DisabledEnum"=w981) -> ()  [unwired: 2 in, 2 out]
                n181 = property on="Capture Exposure Time (s)" class="DigNum (strict)"("DisabledEnum"=w981) -> ()  [unwired: 2 in, 2 out]
              }
              frame True {
              }
            }
            n182 = Get Notifier Status(notifier=w974) -> (notifier out=w973:refnum<notifier>, current notification=w972:T10)  [unwired: 1 in, 3 out]
            n183 = Bundle By Name(cluster=w972, "Line Scan?"=w956, "Actions"=Orca_Flash_Capture_Actions."Idle", "Preview Exposure (s)"=w970, "Capture Exposure (s)"=w970) -> (w969:T10)
            n184 = Select(t=Orca_Flash_Actions."PROGRESSIVE MODE" ("Camera Actions"), s=w956, f=Orca_Flash_Actions."AREA MODE" ("Camera Actions")) -> (s? t:f=w965:T19)
            n185 = call "Orca Flash Messanger.vi"("Notifier Name"=w968, "Camera Actions"=w965) -> ()  [unwired: 9 in, 5 out]
            n186 = Send Notification(notification=w969, notifier=w973) -> ()  [unwired: 1 in, 2 out]
          }
          event Value Change {
            n187 = event-data() -> ("NewVal"=w991:T3)  [unwired: 1 in]
            n188 = Get Notifier Status(notifier=w1000) -> (notifier out=w999:refnum<notifier>, current notification=w998:T10)  [unwired: 1 in, 3 out]
            n189 = Bundle By Name(cluster=w998, "Actions"=Orca_Flash_Capture_Actions."Idle", "Line Scan Mode"=w991) -> (w997:T10)
            n190 = Send Notification(notification=w997, notifier=w999) -> ()  [unwired: 1 in, 2 out]
            n191 = Equal?(x=w991, y=Orca_Flash_Capture_Switch_Line_Scan_Modes."Use Presets") -> (x = y?=w983:bool)
            n192 = Not Equal?(x=w991, y=Orca_Flash_Capture_Switch_Line_Scan_Modes."Automatic") -> (x != y?=w985:bool)
            n193 = Select(t=T8."Enabled" ("Disabled"), s=w983, f=T8."Enabled" ("Disabled")) -> (s? t:f=w993:T8)
            n194 = property on="Line Scanning Presets" class="Ring (strict)"("DisabledEnum"=w993) -> ()  [unwired: 2 in, 2 out]
            n195 = case shown="True" w983 {
              frame False {
              }
              frame True {
                n196 = property on="Line Scanning Presets" class="Ring (strict)"() -> ("Value"=w1003:u16)  [unwired: 2 in, 2 out]
                n197 = property on="Line Scanning Presets" class="Ring (strict)"("Val(Sgnl)"=w1003) -> ()  [unwired: 2 in, 2 out]
              }
            }
            n198 = Select(t=T8."Disabled and Grayed Out" ("Disabled"), s=w985, f=T8."Enabled" ("Disabled")) -> (s? t:f=w984:T8)
            n199 = Select(t=T8."Enabled" ("Disabled"), s=w985, f=T8."Enabled" ("Disabled")) -> (s? t:f=w988:T8)
            n200 = property on="Preview Exposure Time (s)" class="DigNum (strict)"("DisabledEnum"=w984) -> ()  [unwired: 2 in, 2 out]
            n201 = property on="Capture Exposure Time (s)" class="DigNum (strict)"("DisabledEnum"=w984) -> ()  [unwired: 2 in, 2 out]
            n202 = property on="Save As Preset" class="Bool"("DisabledEnum"=w988) -> ()  [unwired: 2 in, 2 out]
            n203 = property on="Line Scan Settings" class="Clust (strict)"("DisabledEnum"=w988) -> ()  [unwired: 2 in, 2 out]
          }
          event "Line Scanning Presets": Value Change {
            n204 = event-data() -> ("CtlRef"=w1013:refnum<vi>)  [unwired: 1 in]
            n205 = control-ref of="This VI"() -> (w1017:refnum<vi>)
            n206 = property class="Ring (strict)"(reference=w1013) -> ("RingText.Text"=w1011:string)  [unwired: 1 in, 2 out]
            n207 = property class="VI"(reference=w1017) -> ("Path"=w1016:path)  [unwired: 1 in, 2 out]
            n208 = Strip Path(path=w1016) -> (stripped path=w1015:path)  [unwired: 1 out]
            n209 = Concatenate Strings(w1011, ".json" ("string")) -> (w1009:string)
            n210 = Build Path(base path=w1015, name or relative path="Orca Flash Capture Manager Line Scan Presets") -> (appended path=w1012:path)
            n211 = Build Path(base path=w1012, name or relative path=w1009) -> (appended path=w1008:path)
            n212 = Read from Text File(file (use dialog)=w1008) -> (text=w1007:string, error out=w1005:errorcluster)  [unwired: 3 in, 2 out]
            n213 = Unflatten From JSON(JSON string=w1007, type and defaults=T4 {"Interline Interval"=0.0, "Offset (V)"=0.0, "Amplitude (V)"=0.0, "Samples Per Channel"=0.0, "Delay (ms)"=0.0} ("Line Scan Settings"), error in (no error)=w1005) -> (value=w1004:T4)  [unwired: 4 in, 1 out]
            n214 = property on="Line Scan Settings" class="Clust (strict)"("Val(Sgnl)"=w1004) -> ()  [unwired: 2 in, 2 out]
          }
          event Value Change {
            # "If you try and set the ILI while the camera is in area mode it gives an error"
            n215 = event-data() -> ("NewVal"=w1035:T4)  [unwired: 1 in]
            n216 = Get Notifier Status(notifier=w1040) -> (current notification=w1039:T10)  [unwired: 1 in, 4 out]
            n217 = Unbundle By Name(w1035) -> ("Offset (V)"=w1029:dbl, "Amplitude (V)"=w1033:dbl, "Samples Per Channel"=w1032:dbl, "Delay (ms)"=w1031:dbl, "Interline Interval"=w1024:dbl)
            n218 = Unbundle By Name(w1039) -> ("Line Scan?"=w1022:bool)
            n219 = To Long Integer(number=w1032) -> (32bit integer=w1030:i32)
            n220 = feedback-in #1(w1024) -> ()
            n221 = feedback #1(0.0) -> (w1023:dbl)
            n222 = Select(t=w1029, s=w1022, f=0.0) -> (s? t:f=w1027:dbl)
            n223 = Not Equal?(x=w1024, y=w1023) -> (x != y?=w1020:bool)
            n224 = Select(t=AO_SCTR_Actions."Update and Run" ("Actions"), s=w1022, f=AO_SCTR_Actions."Stop at Offset" ("Actions")) -> (s? t:f=w1036:T27)
            n225 = call "AO SCTR Messenger.vi"("Notifier Name"=w1034, "Actions"=w1036, "Offset (V)"=w1027, "Amplitude (V)"=w1033, "Samples Per Channel"=w1030, "Start Delay (ms)"=w1031) -> ()  [unwired: 9 in, 1 out]
            n226 = And(x=w1022, y=w1020) -> (x .and. y?=w1021:bool)
            n227 = case shown="True" w1021 {
              tunnel: w1026 -> [_ w1045]
              tunnel: w1024 -> [_ w1044]
              frame False {
              }
              frame True {
                n228 = Bundle By Name(cluster=T17 {"Value"=0.0, "Parameter"=4226016} ("sCMOS Parameter"), "Value"=w1044) -> (w1048:T17)
                n229 = call "Orca Flash Messanger.vi"("Notifier Name"=w1045, "Camera Actions"=Orca_Flash_Actions."SETPARAM", "sCMOS Parameter"=w1048) -> ("sCMOS Parameter"=w1049:T17)  [unwired: 8 in, 4 out]
                n230 = Unbundle By Name(w1049) -> ("Value"=w1043:dbl)
                n231 = property on="Interline Interval" class="DigNum (strict)"("Value"=w1043) -> ()  [unwired: 2 in, 2 out]
              }
            }
          }
          event "Save As Preset": Value Change {
            n232 = event-data() -> ()  [unwired: 1 in, 6 out]
            n233 = control-ref of="This VI"() -> (w1062:refnum<vi>)
            n234 = property class="VI"(reference=w1062) -> ("Path"=w1061:path)  [unwired: 1 in, 2 out]
            n235 = Strip Path(path=w1061) -> (stripped path=w1060:path)  [unwired: 1 out]
            n236 = Build Path(base path=w1060, name or relative path="Orca Flash Capture Manager Line Scan Presets") -> (appended path=w1051:path)
            n237 = call "File Dialog"("start path"=w1051, "prompt"="Save Preset File", "pattern (all files)"="*.json", "pattern label"="JSON") -> ("selected path"=w1056:path, "error out"=w1057:errorcluster)  [unwired: 8 in, 2 out]
            n238 = case shown="No Error" w1057 {
              selector: w1057 -> [_ w1082]
              tunnel: w1056 -> [w1081 _]
              tunnel: [w1075 w1082] -> w1050
              frame No Error {
                n239 = local read "Line Scan Settings"() -> (w1080:T4)
                n240 = Flatten To JSON(anything=w1080) -> (JSON string=w1079:string, 11:w1078:errorcluster)  [unwired: 2 in]
                n241 = Write to Text File(file (use dialog)=w1081, text=w1079, error in=w1078) -> (refnum out=w1077:refnum<file>, error out=w1076:errorcluster)  [unwired: 1 in, 1 out]
                n242 = Close File(refnum=w1077, error in=w1076) -> (error out=w1075:errorcluster)  [unwired: 1 out]
              }
              frame Error {
              }
            }
            n243 = List Folder(path=w1051, pattern="*.json", error in=w1050) -> (filenames=w1054:string[], error out=w1053:errorcluster)  [unwired: 1 in, 2 out]
            n244 = case shown="No Error" w1053 {
              tunnel: w1054 -> [w1069 _]
              tunnel: w1051 -> [w1068 _]
              tunnel: [w1067 string[] []] -> w1052
              frame No Error {
                n245 = for {
                  tunnel: w1069 -> [w1072] mode=indexing
                  tunnel: w1068 -> [w1073]
                  tunnel: [w1070] -> w1067 mode=indexing
                  n246 = Build Path(base path=w1073, name or relative path=w1072) -> (appended path=w1071:path)
                  n247 = call <vilib>:"Get File Extension.vi"("file"=w1071) -> ("filename without extension"=w1070:string)  [unwired: 6 in, 4 out]
                }
              }
              frame Error {
              }
            }
            n248 = property on="Line Scanning Presets" class="Ring (strict)"("Strings []"=w1052) -> ()  [unwired: 2 in, 2 out]
          }
          event "Quit": Value Change {
            n249 = event-data() -> ("NewVal"=w1097:bool)  [unwired: 1 in]
            n250 = Get Notifier Status(notifier=w1096) -> (notifier out=w1095:refnum<notifier>, current notification=w1094:T10)  [unwired: 1 in, 3 out]
            n251 = Bundle By Name(cluster=w1094, "Running?"=FALSE ("Abort"), "Actions"=Orca_Flash_Capture_Actions."Quit") -> (w1088:T10)
            n252 = Send Notification(notification=w1088, notifier=w1095) -> (notifier out=w1092:refnum<notifier>)  [unwired: 1 in, 1 out]
            n253 = Wait on Notification(notifier=w1092, ignore previous (F)=TRUE, timeout in ms (-1)=500) -> (notifier out=w1089:refnum<notifier>)  [unwired: 1 in, 3 out]
            n254 = Send Notification(notification=w1088, notifier=w1089) -> (notifier out=w1086:refnum<notifier>)  [unwired: 1 in, 1 out]
            n255 = Release Notifier(notifier=w1086, force destroy? (F)=TRUE) -> ()  [unwired: 1 in, 3 out]
            n256 = for {
              tunnel: w1084 -> [w1098] mode=indexing
              n257 = call "IMAQ Dispose"("Image"=w1098) -> ()  [unwired: 5 in, 1 out]
            }
          }
        }
      }
      n258 = while {
        tunnel: w219 -> [w249]
        tunnel: w187 -> [w243]
        tunnel: w218 -> [w241]
        tunnel: [FALSE] -> w217
        tunnel: w211 -> [w239]
        tunnel: w181 -> [w237]
        tunnel: w180 -> [w236]
        tunnel: w179 -> [w235]
        tunnel: w178 -> [w234]
        tunnel: [w234] -> w177
        tunnel: w170 -> [w233]
        stop <- w245 stop-if-true
        w231 = u16 0 ("Current Step")
        n259 = Wait on Notification(notifier=w249, ignore previous (F)=TRUE) -> (notifier out=w244:refnum<notifier>, notification=w247:T10)  [unwired: 2 in, 2 out]
        n260 = Unbundle By Name(w247) -> ("Actions"=w242:T11)
        n261 = Bundle By Name(cluster=T20 {"Scan Mode"=enum."Steps Then Cycles", "Current Step"=0, "Current Cycle"=0, "Num of Steps"=0, "Num of Cycles"=0} ("Cycles Steps Tracker"), "Current Step"=w231, "Current Cycle"=w231, "Num of Steps"=w231, "Num of Cycles"=w231, "Scan Mode"="Scan Mode") -> (w238:T20)
        n262 = Equal?(x=w242, y=Orca_Flash_Capture_Actions."Quit") -> (x = y?=w245:bool)
        n263 = while {
          shift-right: [w264] -> _
          shift-left: w242 -> [w265]
          tunnel: w244 -> [w258]
          tunnel: w243 -> [w261]
          tunnel: w242 -> [w260]
          tunnel: w241 -> [w259]
          tunnel: w239 -> [w257]
          shift-right: [w255] -> _
          shift-left: w238 -> [w256]
          tunnel: w237 -> [w254]
          tunnel: w236 -> [w253]
          tunnel: w235 -> [w252]
          tunnel: w234 -> [w251]
          tunnel: w233 -> [w250]
          stop <- w262 stop-if-true
          n264 = case shown="\"Write Metadata\"" w265 {
            selector: w265 -> [_ _ _ w346 _ _ _ _ _ _ _ _ _ _ _]
            tunnel: [Orca_Flash_Capture_Actions."Quit" ("y") Orca_Flash_Capture_Actions."Laser On" ("y") Orca_Flash_Capture_Actions."Laser Off" ("y") w340 Orca_Flash_Capture_Actions."Start Acquisition" ("y") w411 Orca_Flash_Capture_Actions."Write Metadata" ("y") w503 Orca_Flash_Capture_Actions."Camera" ("y") w545 w588 Orca_Flash_Capture_Actions."Setup" ("y") Orca_Flash_Capture_Actions."External Cycle Sync" ("y") w711 Orca_Flash_Capture_Actions."Quit" ("y")] -> w264
            tunnel: [w267 w279 w309 w344 w368 w413 w480 w513 w523 w554 w608 w623 w679 w732 TRUE] -> w262
            tunnel: FALSE -> [w267 w279 w309 w344 w368 w413 w480 w513 w523 w554 w608 w623 w679 w732 _]
            tunnel: w261 -> [_ w272 w306 _ w353 w412 _ _ _ w542 _ _ _ _ _]
            tunnel: w260 -> [_ _ w305 _ w361 w409 w477 w510 _ _ _ _ _ _ _]
            tunnel: w259 -> [_ _ _ w343 _ _ _ _ _ w537 _ _ _ _ _]
            tunnel: w258 -> [_ _ w303 _ w366 w410 w479 w512 _ w546 w595 w615 w677 _ w754]
            tunnel: w257 -> [_ _ w300 _ _ w408 _ _ _ _ _ w614 w678 _ _]
            tunnel: w256 -> [w266 w278 w286 w338 w356 w407 w478 w511 w521 w535 w593 w613 w662 w731 w764]
            tunnel: [w266 w278 w286 w338 w356 w406 w478 w511 w521 w535 w607 w613 w662 w731 w764] -> w255
            tunnel: w254 -> [_ _ _ _ w349 _ _ _ _ _ _ _ _ _ _]
            tunnel: w253 -> [_ _ _ _ w348 _ _ _ _ _ _ _ _ _ _]
            tunnel: w252 -> [_ _ _ _ w347 _ _ _ _ _ _ _ _ _ _]
            tunnel: w251 -> [_ w271 _ _ _ w405 _ _ _ w534 _ _ w663 _ w759]
            tunnel: w250 -> [_ _ w282 _ _ _ _ _ _ _ _ _ _ _ _]
            frame "Idle", Default {
            }
            frame "Live Preview", "Capture" {
              w269 = FALSE ("Camera Running?")
              n265 = call "Orca Flash Messanger.vi"("Notifier Name"=w272, "Camera Actions"=Orca_Flash_Actions."STATUS") -> ("Image Ref"=w273:T5)  [unwired: 9 in, 4 out]
              n266 = Get Notifier Status(notifier=w271) -> (notifier out=w276:refnum<notifier>, current notification=w277:T6)  [unwired: 1 in, 3 out]
              n267 = Bundle By Name(cluster=w277, "Image Ref"=w273, "Cycle Number"=u32 0, "Camera Running?"=w269, "Capture?"=w269) -> (w275:T6)
              n268 = Send Notification(notification=w275, notifier=w276) -> ()  [unwired: 1 in, 2 out]
            }
            frame "Abort" {
              w302 = u16 1 ("Current Cycle")
              w307 = FALSE ("Live Preview")
              n269 = call "Orca Flash Messanger.vi"("Notifier Name"=w306, "Camera Actions"=Orca_Flash_Actions."IDLE") -> ()  [unwired: 9 in, 5 out]
              n270 = local write "Live Preview"(w307) -> ()
              n271 = local write "Capture"(w307) -> ()
              n272 = Equal?(x=Orca_Flash_Capture_Actions."Capture", y=w305) -> (x = y?=w299:bool)
              n273 = Get Notifier Status(notifier=w303) -> (current notification=w281:T10)  [unwired: 1 in, 4 out]
              n274 = local write "Current Cycle"(w302) -> ()
              n275 = local write "Current Step"(w302) -> ()
              n276 = Unbundle By Name(w281) -> ("Init Z Position (µm)"=w301:dbl)
              n277 = Obtain Notifier(name (unnamed)="WFDC External Sync", notification data type=T22 {"Cycle Sync"=enum."Pause Requested", "Z Offset"=0.0, "WFDC Status"=enum."Idle"} ("WFDC External Sync"), create if not found? (T)=FALSE) -> (notifier out=w293:refnum<notifier>, error out=w298:errorcluster)  [unwired: 1 in, 1 out]
              n278 = Get Notifier Status(notifier=w293, error in (no error)=w298) -> (notifier out=w288:refnum<notifier>, current notification=w287:T22, error out=w297:errorcluster)  [unwired: 2 out]
              n279 = Unbundle By Name(w287) -> ("WFDC Status"=w285:T21)
              n280 = Unbundle By Name(w297) -> ("status"=w296:bool)
              n281 = Not Equal?(x=WFDC_Status."DC Active", y=w285) -> (x != y?=w295:bool)
              n282 = Equal?(x=w285, y=WFDC_Status."Error") -> (x = y?=w283:bool)
              n283 = Or(x=w295, y=w296) -> (x .or. y?=w289:bool)
              n284 = case shown="True" w299 {
                tunnel: w301 -> [_ w318]
                tunnel: w300 -> [_ w317]
                tunnel: w289 -> [_ w316]
                tunnel: w288 -> [_ w315]
                tunnel: w287 -> [_ w314]
                tunnel: w283 -> [_ w312]
                tunnel: w282 -> [_ w311]
                frame False {
                }
                frame True {
                  n285 = case shown="False" w316 {
                    tunnel: w318 -> [_ w336]
                    tunnel: w317 -> [_ w335]
                    tunnel: w315 -> [w329 _]
                    tunnel: w314 -> [w328 _]
                    frame False {
                      n286 = Bundle By Name(cluster=w328, "Z Offset"=0.0) -> (w330:T22)
                      n287 = Send Notification(notification=w330, notifier=w329) -> (notifier out=w325:refnum<notifier>)  [unwired: 1 in, 1 out]
                      n288 = Release Notifier(notifier=w325, force destroy? (F)=FALSE) -> ()  [unwired: 1 in, 3 out]
                    }
                    frame True {
                      n289 = Build Array(w336) -> (w331:dbl[])
                      n290 = call "Stages Messenger.vi"("Stage Notifier Name"=w335, "Actions"=Stage_Actions."MOVE", "Setpoint"=w331, "Axis"=bool[] [TRUE], "Exit While Busy?"=FALSE) -> ()  [unwired: 7 in, 4 out]
                    }
                  }
                  n291 = case shown="True" "Email Alerts" {
                    tunnel: w312 -> [_ w321]
                    tunnel: w311 -> [_ w319]
                    frame False {
                    }
                    frame True {
                      n292 = Select(t="Acquisition Error - Abort", s=w321, f="Acquisition Finished") -> (s? t:f=w320:string)
                      n293 = call "SMTP Email Alerts Messenger.vi"("Notifier Name"=w319, "Actions"=SMTP_Email_Alerts_Actions."Send Message", "Subject"=w320, "Body Text"=w320) -> ()  [unwired: 12 in]
                    }
                  }
                }
              }
            }
            frame "Laser On", "Laser Off" {
              n294 = Equal?(x=w346, y=Orca_Flash_Capture_Actions."Laser On") -> (x = y?=w337:bool)
              n295 = call "AOTF Messenger.vi"("AOTF Notifier Name"=w343, "AOTF Action"=AOTF_Actions."Blank", "Beam Blank"=w337) -> ()  [unwired: 8 in, 5 out]
              n296 = Select(t=Orca_Flash_Capture_Actions."Set Exposure Time" ("y"), s=w337, f=Orca_Flash_Capture_Actions."Quit" ("y")) -> (s? t:f=w340:T11)
            }
            frame "Set Exposure Time" {
              # "Frame Rate (Hz)"
              n297 = Get Notifier Status(notifier=w366) -> (current notification=w362:T10)  [unwired: 1 in, 4 out]
              n298 = Unbundle By Name(w362) -> ("Line Scan?"=w351:bool, "Line Scan Mode"=w350:T3, "Capture Exposure (s)"=w357:dbl, "Preview Exposure (s)"=w358:dbl)
              n299 = Equal?(x=w361, y=Orca_Flash_Capture_Actions."Capture") -> (x = y?=w359:bool)
              n300 = Select(t=w357, s=w359, f=w358) -> (s? t:f=w355:dbl)
              n301 = case shown="True" w351 {
                tunnel: w355 -> [w370 w379]
                tunnel: [w370 w376] -> w354
                tunnel: w353 -> [w369 w378]
                tunnel: [w369 w375] -> w352
                tunnel: w350 -> [_ w374]
                tunnel: w349 -> [_ w373]
                tunnel: w348 -> [_ w372]
                tunnel: w347 -> [_ w371]
                frame False {
                  # "Exposure Time (s)"
                }
                frame True {
                  n302 = To Double Precision Float(number="Number of Lines") -> (double precision float=w377:dbl)
                  n303 = case shown="\"Automatic\"" w374 {
                    tunnel: w379 -> [_ w404]
                    tunnel: w378 -> [w385 w403]
                    tunnel: w377 -> [w383 w402]
                    tunnel: [w381 w401] -> w376
                    tunnel: [w384 w400] -> w375
                    tunnel: w373 -> [_ w393]
                    tunnel: w372 -> [_ w390]
                    tunnel: w371 -> [_ w389]
                    frame Default {
                      n304 = call "Orca Flash Messanger.vi"("Notifier Name"=w385, "Camera Actions"=Orca_Flash_Actions."GETPARAM", "sCMOS Parameter"=T17 {"Value"=0.0, "Parameter"=4226016}) -> ("Notifier Name Dup"=w384:string, "sCMOS Parameter"=w388:T17)  [unwired: 8 in, 3 out]
                      n305 = Unbundle By Name(w388) -> ("Value"=w382:dbl)
                      n306 = Multiply(x=w382, y=w383) -> (x*y=w381:dbl)
                    }
                    frame "Automatic" {
                      n307 = call "Orca Flash Capture Set Interline Interval.vi"("Camera Notifier Name"=w403, "Frame Rate (Hz)"=w404) -> ("Camera Notifier Name (Dup)"=w400:string, "Interline Interval (s)"=w399:dbl)  [unwired: 12 in]
                      n308 = Multiply(x=w399, y=w402) -> (x*y=w401:dbl)
                      n309 = call "Orca Flash Capture Set Auto Waveform.vi"("Interline Interval"=w399, "Filter Index"="Current Filter", "Waveform Parameters"=w390, "Filter Offsets"=w389) -> ("Offset (V)"=w397:dbl, "Amplitude (V)"=w396:dbl, "Samples per Channel"=w395:i32, "Delay (ms)"=w394:dbl, "Line Scan Settings"=w392:T4)  [unwired: 7 in]
                      n310 = local write "Line Scan Settings"(w392) -> ()
                      n311 = call "AO SCTR Messenger.vi"("Notifier Name"=w393, "Actions"=AO_SCTR_Actions."Update and Run", "Offset (V)"=w397, "Amplitude (V)"=w396, "Samples Per Channel"=w395, "Start Delay (ms)"=w394) -> ()  [unwired: 9 in, 1 out]
                    }
                  }
                }
              }
              n312 = Bundle By Name(cluster=T17 {"Value"=0.0, "Parameter"=2049184} ("sCMOS Parameter"), "Value"=w354) -> (w365:T17)
              n313 = call "Orca Flash Messanger.vi"("Notifier Name"=w352, "Camera Actions"=Orca_Flash_Actions."SETPARAM", "sCMOS Parameter"=w365) -> ()  [unwired: 8 in, 5 out]
            }
            frame "Start Acquisition" {
              n314 = case shown="\"Capture\"" w409 {
                tunnel: w412 -> [_ w416 _]
                tunnel: [Orca_Flash_Capture_Actions."Quit" ("y") Orca_Flash_Capture_Actions."Quit" ("y") Orca_Flash_Capture_Actions."Update SubFolder" ("y")] -> w411
                tunnel: w410 -> [_ _ w451]
                tunnel: w408 -> [_ _ w443]
                tunnel: w407 -> [w414 w417 w439]
                tunnel: [w414 w417 w438] -> w406
                tunnel: w405 -> [_ _ w431]
                frame Default {
                }
                frame "Live Preview" {
                  n315 = call "Orca Flash Messanger.vi"("Notifier Name"=w416, "Camera Actions"=Orca_Flash_Actions."PREVIEW") -> ()  [unwired: 9 in, 5 out]
                }
                frame "Capture" {
                  w437 = sgl 0.0 ("Cycle")
                  n316 = Get Notifier Status(notifier=w431) -> (notifier out=w435:refnum<notifier>, current notification=w434:T6)  [unwired: 1 in, 3 out]
                  n317 = Bundle By Name(cluster=w434, "Capture?"=TRUE) -> (w433:T6)
                  n318 = call "Stages Messenger.vi"("Stage Notifier Name"=w443, "Actions"=Stage_Actions."Get Position") -> ("Positions"=w446:dbl[])  [unwired: 10 in, 3 out]
                  n319 = Send Notification(notification=w433, notifier=w435) -> ()  [unwired: 1 in, 2 out]
                  n320 = Index Array(array=w446, index=0) -> (element=w444:dbl)
                  n321 = local write "Z Step"(w437) -> ()
                  n322 = local write "Cycle"(w437) -> ()
                  n323 = local write "Frame"(u32 0 ("Frame")) -> ()
                  n324 = Get Notifier Status(notifier=w451) -> (notifier out=w448:refnum<notifier>, current notification=w449:T10)  [unwired: 1 in, 3 out]
                  n325 = Bundle By Name(cluster=w449, "Init Z Position (µm)"=w444) -> (w440:T10)
                  n326 = Unbundle By Name(w440) -> ("Cycles"=w441:u16, "No. of Z Steps"=w442:u16)
                  n327 = Send Notification(notification=w440, notifier=w448) -> ()  [unwired: 1 in, 2 out]
                  n328 = Bundle By Name(cluster=w439, "Num of Cycles"=w441, "Num of Steps"=w442) -> (w438:T20)
                  n329 = Obtain Notifier(name (unnamed)="WFDC External Sync", notification data type=T22 {"Cycle Sync"=enum."Pause Requested", "Z Offset"=0.0, "WFDC Status"=enum."Idle"} ("WFDC External Sync"), create if not found? (T)=FALSE) -> (notifier out=w429:refnum<notifier>, error out=w430:errorcluster)  [unwired: 1 in, 1 out]
                  n330 = Get Notifier Status(notifier=w429, error in (no error)=w430) -> (notifier out=w424:refnum<notifier>, current notification=w423:T22, error out=w422:errorcluster)  [unwired: 2 out]
                  n331 = Unbundle By Name(w423) -> ("WFDC Status"=w425:T21)
                  n332 = case shown="\"Error\"" w425 {
                    tunnel: w424 -> [w454 w459]
                    tunnel: w423 -> [_ w458]
                    tunnel: w422 -> [w453 w456]
                    tunnel: [w454 w457] -> w420
                    tunnel: [w453 w455] -> w421
                    frame Default {
                    }
                    frame "Error" {
                      n333 = Two Button Dialog(message="Reset Wide Field Drift Correction error?", 1:"No" ("F button name (\"Cancel\")"), 2:"Yes" ("T button name (\"OK\")")) -> (T button?=w463:bool)
                      n334 = case shown="True" w463 {
                        tunnel: w459 -> [w465 w470]
                        tunnel: w458 -> [_ w472]
                        tunnel: [w465 w468] -> w457
                        tunnel: w456 -> [w464 w467]
                        tunnel: [w464 w466] -> w455
                        frame False {
                        }
                        frame True {
                          n335 = Bundle By Name(cluster=w472, "WFDC Status"=WFDC_Status."Idle") -> (w469:T22)
                          n336 = Send Notification(notification=w469, notifier=w470, error in (no error)=w467) -> (notifier out=w468:refnum<notifier>, error out=w466:errorcluster)
                        }
                      }
                    }
                  }
                  n337 = case shown="No Error" w421 {
                    tunnel: w420 -> [w452 _]
                    frame No Error {
                      n338 = Release Notifier(notifier=w452) -> ()  [unwired: 2 in, 3 out]
                    }
                    frame Error {
                    }
                  }
                }
              }
            }
            frame "Update SubFolder" {
              n339 = Equal?(x=w477, y=Orca_Flash_Capture_Actions."Capture") -> (x = y?=w475:bool)
              n340 = And(x=w475, y="Auto Update Subfolder") -> (x .and. y?=w473:bool)
              n341 = case shown="True" w473 {
                tunnel: w479 -> [w486 w502]
                frame False {
                  n342 = Get Notifier Status(notifier=w486) -> (notifier out=w485:refnum<notifier>, current notification=w483:T10)  [unwired: 1 in, 3 out]
                  n343 = Unbundle By Name(w483) -> ("Base Path"=w482:path)
                  n344 = Bundle By Name(cluster=w483, "Save Path"=w482) -> (w484:T10)
                  n345 = Send Notification(notification=w484, notifier=w485) -> ()  [unwired: 1 in, 2 out]
                }
                frame True {
                  n346 = Get Notifier Status(notifier=w502) -> (notifier out=w490:refnum<notifier>, current notification=w489:T10)  [unwired: 1 in, 3 out]
                  n347 = feedback #2(u32 0) -> (w492:u32)
                  n348 = Unbundle By Name(w489) -> ("Base Path"=w501:path)
                  n349 = Increment(x=w492) -> (x+1=w491:u32)
                  n350 = feedback-in #2(w491) -> ()
                  n351 = Format Into String(format string="%03d", w491) -> (resulting string=w493:string)  [unwired: 2 in, 1 out]
                  n352 = Strip Path(path=w501) -> (stripped path=w500:path, name=w498:string)
                  n353 = Concatenate Strings("Subfolder Name", w493) -> (w496:string)
                  n354 = Build Path(base path=w500, name or relative path=w496) -> (appended path=w499:path)
                  n355 = Build Path(base path=w499, name or relative path=w498) -> (appended path=w488:path)
                  n356 = Bundle By Name(cluster=w489, "Save Path"=w488) -> (w487:T10)
                  n357 = Send Notification(notification=w487, notifier=w490) -> ()  [unwired: 1 in, 2 out]
                }
              }
            }
            frame "Write Metadata" {
              n358 = Equal?(x=w510, y=Orca_Flash_Capture_Actions."Capture") -> (x = y?=w508:bool)
              n359 = case shown="False" w508 {
                tunnel: w512 -> [_ w520]
                tunnel: [errorcluster {"status"=FALSE, "code"=0, "source"=""} ("Write Errror") w515] -> w507
                frame False {
                }
                frame True {
                  n360 = Get Notifier Status(notifier=w520) -> (current notification=w519:T10)  [unwired: 1 in, 4 out]
                  n361 = Unbundle By Name(w519) -> ("Save Path"=w518:path)
                  n362 = call "Write Device Metadata.vi"("File Path"=w518) -> ("File Path (Dup)"=w517:path, "Write Errror"=w516:errorcluster)  [unwired: 13 in]
                  n363 = call "Write Microscope Metadata.vi"("File Path"=w517, "Error In"=w516) -> ("Write Errror"=w515:errorcluster)  [unwired: 12 in, 1 out]
                }
              }
              n364 = Unbundle By Name(w507) -> ("status"=w506:bool)
              n365 = Select(t=Orca_Flash_Capture_Actions."Abort" ("y"), s=w506, f=Orca_Flash_Capture_Actions."Setup" ("y")) -> (s? t:f=w503:T11)
            }
            frame "Setup" {
              # "Change lasers here"
            }
            frame "Camera" {
              n366 = Get Notifier Status(notifier=w546) -> (notifier out=w553:refnum<notifier>, current notification=w538:T10)  [unwired: 1 in, 3 out]
              n367 = Unbundle By Name(w538) -> ("Lasers Lines"=w539:string[])
              n368 = for {
                tunnel: w539 -> [w559] mode=indexing
                tunnel: w537 -> [w558]
                tunnel: [w555] -> w536
                stop <- w556 stop-if-true
                n369 = call "AOTF Messenger.vi"("AOTF Notifier Name"=w558, "AOTF Action"=AOTF_Actions."Status", "Wavelength (nm)"=w559) -> ("Wavelength (nm) Out"=w555:string, "Line On/Off Out"=w556:bool)  [unwired: 8 in, 3 out]
              }
              n370 = Unbundle By Name(w535) -> ("Current Cycle"=w544:u16, "Current Step"=w543:u16)
              n371 = Unbundle By Name(w538) -> ("Save Path"=w549:path, "Frames"=w540:u32)
              n372 = Get Notifier Status(notifier=w534) -> (notifier out=w533:refnum<notifier>, current notification=w532:T6)  [unwired: 1 in, 3 out]
              n373 = Bundle By Name(cluster=w532, "Camera Running?"=TRUE) -> (w530:T6)
              n374 = call "Orca Flash Capture File Name Increment.vi"("Step"=w543, "Cycle"=w544, "Laser Line"=w536, "Path In"=w549) -> ("Path Out"=w550:path)  [unwired: 7 in]
              n375 = call "Orca Flash Messanger.vi"("Notifier Name"=w542, "Camera Actions"=Orca_Flash_Actions."Record Settings", "Path"=w550, "# of frames"=w540) -> ("Notifier Name Dup"=w552:string)  [unwired: 7 in, 4 out]
              n376 = call "Orca Flash Messanger.vi"("Notifier Name"=w552, "Camera Actions"=Orca_Flash_Actions."RECORD") -> ("Notifier Name Dup"=w547:string, "Image Ref"=w541:T5)  [unwired: 9 in, 3 out]
              n377 = Send Notification(notification=w530, notifier=w533) -> (notifier out=w529:refnum<notifier>)  [unwired: 1 in, 1 out]
              n378 = while {
                tunnel: w547 -> [w581]
                tunnel: [w578] -> w545
                tunnel: w553 -> [w567]
                tunnel: w541 -> [w566]
                tunnel: [w560] -> w525
                tunnel: w529 -> [w560]
                stop <- w574 stop-if-true
                n379 = Get Notifier Status(notifier=w567) -> (current notification=w580:T10)  [unwired: 1 in, 4 out]
                n380 = Unbundle By Name(w580) -> ("Running?"=w573:bool)
                n381 = Wait (ms)(milliseconds to wait=u32 25) -> ()  [unwired: 1 out]
                n382 = call "IMAQ Read Custom Data"("Key"="Image Data", "Image"=w566) -> ("Custom Data Out"=w564:string)  [unwired: 7 in, 2 out]
                n383 = Unflatten From JSON(JSON string=w564, type and defaults=T28 {"Frame"=0, "Sensor Height"=0, "Sensor Width"=0, "ROI Height"=0, "ROI Width"=0, "ROI Enable?"=FALSE, "Bit per Pixel"=0} ("Camera IMAQ Key Info")) -> (value=w562:T28)  [unwired: 5 in, 1 out]
                n384 = Not(x=w573) -> (.not. x?=w577:bool)
                n385 = Unbundle By Name(w562) -> ("Frame"=→"Frame" →"Current Frame":u32)
                n386 = Select(t=Orca_Flash_Actions."STATUS" ("Camera Actions"), s=w573, f=Orca_Flash_Actions."IDLE") -> (s? t:f=w568:T19)
                n387 = call "Orca Flash Messanger.vi"("Notifier Name"=w581, "Camera Actions"=w568) -> ("Running?"=w576:bool)  [unwired: 9 in, 4 out]
                n388 = Not(x=w576) -> (.not. x?=w575:bool)
                n389 = Or(x=w577, y=w575) -> (x .or. y?=w574:bool)
                n390 = Select(t=Orca_Flash_Capture_Actions."Switch" ("y"), s=w573, f=Orca_Flash_Capture_Actions."Abort") -> (s? t:f=w578:T11)
              }
              n391 = Get Notifier Status(notifier=w525) -> (notifier out=w524:refnum<notifier>, current notification=w526:T6)  [unwired: 1 in, 3 out]
              n392 = Bundle By Name(cluster=w526, "Camera Running?"=FALSE) -> (w528:T6)
              n393 = Send Notification(notification=w528, notifier=w524) -> ()  [unwired: 1 in, 2 out]
            }
            frame "Switch" {
              n394 = Get Notifier Status(notifier=w595) -> (current notification=w594:T10)  [unwired: 1 in, 4 out]
              n395 = Unbundle By Name(w594) -> ("Cycles"=w590:u16, "No. of Z Steps"=w591:u16)
              n396 = Bundle By Name(cluster=w593, "Num of Cycles"=w590, "Num of Steps"=w591) -> (w592:T20)
              n397 = Unbundle By Name(w592) -> ("Current Cycle"=w604:u16, "Num of Cycles"=w603:u16, "Current Step"=w602:u16, "Num of Steps"=w601:u16)
              n398 = Increment(x=w604) -> (x+1=w587:u16)
              n399 = Increment(x=w602) -> (x+1=w586:u16)
              n400 = To Single Precision Float(number=w587) -> (single precision float=w600:sgl)
              n401 = To Single Precision Float(number=w603) -> (single precision float=w599:sgl)
              n402 = To Single Precision Float(number=w586) -> (single precision float=w598:sgl)
              n403 = To Single Precision Float(number=w601) -> (single precision float=w597:sgl)
              n404 = Divide(x=w600, y=w599) -> (x/y=→"Cycle":sgl)
              n405 = Divide(x=w598, y=w597) -> (x/y=→"Z Step":sgl)
              n406 = call "Orca Flash Capture Scan Counter Cycles Steps.vi"("Cycles Steps Tracker"=w592) -> ("Cycles Steps Tracker Out"=w607:T20, "Change Cycle?"=w584:bool, "Done?"=w606:bool)  [unwired: 8 in]
              n407 = Select(t=Orca_Flash_Capture_Actions."Cycle" ("y"), s=w584, f=Orca_Flash_Capture_Actions."Step") -> (s? t:f=w582:T11)
              n408 = Select(t=Orca_Flash_Capture_Actions."Abort" ("y"), s=w606, f=w582) -> (s? t:f=w588:T11)
              n409 = case shown="Default" w588 {
                tunnel: w587 -> [_ w610 _]
                tunnel: w586 -> [_ _ w612]
                frame Default {
                }
                frame "Cycle" {
                  n410 = Increment(x=w610) -> (x+1=→"Current Cycle":u16)
                }
                frame "Step" {
                  n411 = Increment(x=w612) -> (x+1=→"Current Step":u16)
                }
              }
            }
            frame "Step" {
              n412 = Get Notifier Status(notifier=w615) -> (current notification=w616:T10)  [unwired: 1 in, 4 out]
              n413 = Unbundle By Name(w616) -> ("Z Step Size (µm)"=w622:dbl, "No. of Z Steps"=w619:u16)
              n414 = Less?(x=w619, y=u16 2) -> (x < y?=w620:bool)
              n415 = Equal To 0?(x=w622) -> (x = 0?=w617:bool)
              n416 = Or(x=w617, y=w620) -> (x .or. y?=w618:bool)
              n417 = case shown="False" w618 {
                tunnel: w614 -> [w642 _]
                tunnel: w622 -> [w641 _]
                tunnel: w613 -> [w628 _]
                frame False {
                  n418 = Unbundle By Name(w628) -> ("Current Step"=w627:u16)
                  n419 = Obtain Notifier(name (unnamed)="WFDC External Sync", notification data type=T22 {"Cycle Sync"=enum."Pause Requested", "Z Offset"=0.0, "WFDC Status"=enum."Idle"} ("WFDC External Sync"), create if not found? (T)=FALSE) -> (notifier out=w634:refnum<notifier>, error out=w640:errorcluster)  [unwired: 1 in, 1 out]
                  n420 = Get Notifier Status(notifier=w634, error in (no error)=w640) -> (notifier out=w629:refnum<notifier>, current notification=w626:T22, error out=w639:errorcluster)  [unwired: 2 out]
                  n421 = Unbundle By Name(w626) -> ("WFDC Status"=w635:T21)
                  n422 = Unbundle By Name(w639) -> ("status"=w638:bool)
                  n423 = Not Equal?(x=WFDC_Status."DC Active", y=w635) -> (x != y?=w637:bool)
                  n424 = Or(x=w637, y=w638) -> (x .or. y?=w630:bool)
                  n425 = case shown="False" w630 {
                    tunnel: w642 -> [_ w658]
                    tunnel: w641 -> [w649 w657]
                    tunnel: w629 -> [w646 _]
                    tunnel: w627 -> [w651 _]
                    tunnel: w626 -> [w650 _]
                    tunnel: [u32 350 ("milliseconds to wait") u32 100 ("milliseconds to wait")] -> w625
                    frame False {
                      n426 = To Double Precision Float(number=w651) -> (double precision float=w648:dbl)
                      n427 = Multiply(x=w649, y=w648) -> (x*y=w647:dbl)
                      n428 = Bundle By Name(cluster=w650, "Z Offset"=w647) -> (w645:T22)
                      n429 = Send Notification(notification=w645, notifier=w646) -> (notifier out=w643:refnum<notifier>)  [unwired: 1 in, 1 out]
                      n430 = Release Notifier(notifier=w643) -> ()  [unwired: 2 in, 3 out]
                    }
                    frame True {
                      n431 = Build Array(w657) -> (w656:dbl[])
                      n432 = call "Stages Messenger.vi"("Stage Notifier Name"=w658, "Actions"=Stage_Actions."MVR", "Setpoint"=w656, "Axis"=bool[] [TRUE], "Exit While Busy?"=FALSE) -> ()  [unwired: 7 in, 4 out]
                    }
                  }
                  n433 = Wait (ms)(milliseconds to wait=w625) -> ()  [unwired: 1 out]
                }
                frame True {
                }
              }
            }
            frame "Cycle" {
              n434 = Unbundle By Name(w662) -> ("Scan Mode"=w661:T2, "Current Cycle"=w664:u16)
              n435 = Equal?(x=Orca_Flash_Switch_Cycles_Steps."Cycles Then Steps", y=w661) -> (x = y?=w659:bool)
              n436 = Get Notifier Status(notifier=w677) -> (current notification=w676:T10)  [unwired: 1 in, 4 out]
              n437 = Get Notifier Status(notifier=w663) -> (notifier out=w667:refnum<notifier>, current notification=w666:T6)  [unwired: 1 in, 3 out]
              n438 = Bundle By Name(cluster=w666, "Cycle Number"=w664) -> (w665:T6)
              n439 = Unbundle By Name(w676) -> ("Init Z Position (µm)"=w668:dbl, "Z Step Size (µm)"=w672:dbl, "No. of Z Steps"=w671:u16)
              n440 = Send Notification(notification=w665, notifier=w667) -> ()  [unwired: 1 in, 2 out]
              n441 = Equal To 0?(x=w672) -> (x = 0?=w675:bool)
              n442 = Less?(x=w671, y=u16 2) -> (x < y?=w674:bool)
              n443 = Compound Arithmetic op=OR(w675, w674, w659) -> (w670:bool)
              n444 = case shown="False" w670 {
                tunnel: w678 -> [w681 _]
                tunnel: w668 -> [w683 _]
                frame False {
                  n445 = Obtain Notifier(name (unnamed)="WFDC External Sync", notification data type=T22 {"Cycle Sync"=enum."Pause Requested", "Z Offset"=0.0, "WFDC Status"=enum."Idle"} ("WFDC External Sync"), create if not found? (T)=FALSE) -> (notifier out=w689:refnum<notifier>, error out=w695:errorcluster)  [unwired: 1 in, 1 out]
                  n446 = Get Notifier Status(notifier=w689, error in (no error)=w695) -> (notifier out=w684:refnum<notifier>, current notification=w682:T22, error out=w694:errorcluster)  [unwired: 2 out]
                  n447 = Unbundle By Name(w682) -> ("WFDC Status"=w690:T21)
                  n448 = Unbundle By Name(w694) -> ("status"=w693:bool)
                  n449 = Not Equal?(x=WFDC_Status."DC Active", y=w690) -> (x != y?=w692:bool)
                  n450 = Or(x=w692, y=w693) -> (x .or. y?=w685:bool)
                  n451 = case shown="True" w685 {
                    tunnel: w684 -> [w699 _]
                    tunnel: w683 -> [_ w704]
                    tunnel: w682 -> [w698 _]
                    tunnel: w681 -> [_ w703]
                    tunnel: [u32 350 ("milliseconds to wait") u32 100 ("milliseconds to wait")] -> w680
                    frame False {
                      n452 = Bundle By Name(cluster=w698, "Z Offset"=0.0) -> (w701:T22)
                      n453 = Send Notification(notification=w701, notifier=w699) -> (notifier out=w700:refnum<notifier>)  [unwired: 1 in, 1 out]
                      n454 = Release Notifier(notifier=w700) -> ()  [unwired: 2 in, 3 out]
                    }
                    frame True {
                      n455 = Build Array(w704) -> (w705:dbl[])
                      n456 = call "Stages Messenger.vi"("Stage Notifier Name"=w703, "Actions"=Stage_Actions."MOVE", "Setpoint"=w705, "Axis"=bool[] [TRUE], "Exit While Busy?"=FALSE) -> ()  [unwired: 7 in, 4 out]
                    }
                  }
                  n457 = Wait (ms)(milliseconds to wait=w680) -> ()  [unwired: 1 out]
                }
                frame True {
                }
              }
            }
            frame "External Cycle Sync" {
              n458 = Obtain Notifier(name (unnamed)="WFDC External Sync", notification data type=T22 {"Cycle Sync"=enum."Pause Requested", "Z Offset"=0.0, "WFDC Status"=enum."Idle"} ("WFDC External Sync"), create if not found? (T)=FALSE) -> (notifier out=w727:refnum<notifier>, error out=w730:errorcluster)  [unwired: 1 in, 1 out]
              n459 = Get Notifier Status(notifier=w727, error in (no error)=w730) -> (notifier out=w716:refnum<notifier>, current notification=w715:T22, error out=w729:errorcluster)  [unwired: 2 out]
              n460 = Unbundle By Name(w729) -> ("status"=w723:bool)
              n461 = Unbundle By Name(w715) -> ("WFDC Status"=w714:T21, "Cycle Sync"=w722:T23)
              n462 = Not(x=w723) -> (.not. x?=w718:bool)
              n463 = Equal?(x=WFDC_Status."Error", y=w714) -> (x = y?=w710:bool)
              n464 = Equal?(x=WFDC_Status."DC Active", y=w714) -> (x = y?=w720:bool)
              n465 = Equal?(x=w722, y=WFDC_Cycle_Pause."Pause Requested") -> (x = y?=w719:bool)
              n466 = Compound Arithmetic op=AND(w720, w719, w718) -> (w717:bool)
              n467 = case shown="True" w717 {
                tunnel: w716 -> [_ w740]
                tunnel: w715 -> [_ w742]
                frame False {
                }
                frame True {
                  n468 = Bundle By Name(cluster=w742, "Cycle Sync"=WFDC_Cycle_Pause."Paused") -> (w739:T22)
                  n469 = Send Notification(notification=w739, notifier=w740) -> (notifier out=w738:refnum<notifier>)  [unwired: 1 in, 1 out]
                  n470 = while {
                    tunnel: w738 -> [w753]
                    tunnel: [w744] -> w735
                    tunnel: [w743] -> w737
                    i -> [w749]
                    stop <- w745 stop-if-true
                    n471 = Get Notifier Status(notifier=w753) -> (notifier out=w744:refnum<notifier>, current notification=w743:T22)  [unwired: 1 in, 3 out]
                    n472 = Greater?(x=w749, y=15000) -> (0:w746:bool)
                    n473 = Unbundle By Name(w743) -> ("Cycle Sync"=w752:T23)
                    n474 = Equal?(x=w752, y=WFDC_Cycle_Pause."Resume Requested") -> (x = y?=w747:bool)
                    n475 = Or(x=w747, y=w746) -> (x .or. y?=w745:bool)
                    n476 = Wait (ms)(milliseconds to wait=u32 1) -> ()  [unwired: 1 out]
                  }
                  n477 = Bundle By Name(cluster=w737, "Cycle Sync"=WFDC_Cycle_Pause."Resumed") -> (w734:T22)
                  n478 = Send Notification(notification=w734, notifier=w735) -> (notifier out=w733:refnum<notifier>)  [unwired: 1 in, 1 out]
                  n479 = Release Notifier(notifier=w733) -> ()  [unwired: 2 in, 3 out]
                }
              }
              n480 = Select(t=Orca_Flash_Capture_Actions."Abort" ("y"), s=w710, f=Orca_Flash_Capture_Actions."Setup" ("y")) -> (s? t:f=w711:T11)
            }
            frame "Quit" {
              w763 = FALSE ("Capture?")
              n481 = Get Notifier Status(notifier=w754) -> (notifier out=w758:refnum<notifier>, current notification=w757:T10)  [unwired: 1 in, 3 out]
              n482 = Bundle By Name(cluster=w757, "Running?"=FALSE) -> (w755:T10)
              n483 = Send Notification(notification=w755, notifier=w758) -> ()  [unwired: 1 in, 2 out]
              n484 = Get Notifier Status(notifier=w759) -> (notifier out=w762:refnum<notifier>, current notification=w761:T6)  [unwired: 1 in, 3 out]
              n485 = Bundle By Name(cluster=w761, "Camera Running?"=w763, "Capture?"=w763) -> (w760:T6)
              n486 = Send Notification(notification=w760, notifier=w762) -> ()  [unwired: 1 in, 2 out]
            }
          }
        }
      }
      n487 = local write "Quit"(w217) -> ()
      n488 = Release Notifier(notifier=w177) -> ()  [unwired: 2 in, 3 out]
    }
    frame Error {
      n489 = Release Notifier(notifier=w1101) -> (error out=w1100:errorcluster)  [unwired: 2 in, 2 out]
      n490 = for {
        tunnel: w1099 -> [w1106] mode=indexing
        n491 = call "IMAQ Dispose"("Image"=w1106) -> ()  [unwired: 5 in, 1 out]
      }
      n492 = Unbundle By Name(w1100) -> ("source"=w1103:string)
      n493 = Concatenate Strings("4Pi Capture Manager could not start.", "\r", w1103) -> (w1102:string)
      n494 = One Button Dialog(message=w1102) -> ()  [unwired: 1 in, 1 out]
    }
  }
  n495 = control-ref of="This VI"() -> (w106:refnum<vi>)
  n496 = property class="VI"(reference=w106) -> (reference out=w115:refnum<vi>, "Panel"=w107:refnum<vi>)  [unwired: 1 in, 1 out]
  n497 = property class="Pnl"(reference=w107) -> ("Decos[]"=w105:refnum<vi>[], "Panes[]"=w111:refnum<vi>[])  [unwired: 1 in, 2 out]
  n498 = Array Size(array=w105) -> (size(s)=w103:i32)
  n499 = Decrement(x=w103) -> (x-1=w104:i32)
  n500 = Index Array(array=w111, index=0) -> (element=w110:refnum<vi>)
  n501 = Index Array(array=w105, index=w104) -> (element=w113:refnum<vi>)
  n502 = property class="VI"(reference=w115) -> (reference out=w117:refnum<vi>, "Front Panel.PanelBounds"=w118:T30)  [unwired: 1 in, 1 out]
  n503 = property class="Decor"(reference=w113) -> ("Bounds"=w116:T31)  [unwired: 1 in, 2 out]
  n504 = property class="Pane"(reference=w110, "Origin"=T13 {"Horizontal"=0, "Vertical"=0}, "HorizScrollbarVisibility"=w114, "VertScrollbarVisibility"=w114) -> ()  [unwired: 1 in, 2 out]
  n505 = Unbundle By Name(w116) -> ("Width"=w121:u32, "Height"=w124:u32)
  n506 = control-ref of="Quit"() -> (w108:refnum<vi>)
  n507 = To Word Integer(number=w121) -> (16bit integer=w123:i16)
  n508 = To Word Integer(number=w124) -> ()  [unwired: 1 out]
  n509 = property class="Bool (strict)"(reference=w108) -> ("Height"=w126:u32, "Top"=w127:i32)  [unwired: 1 in, 2 out]
  n510 = Unbundle By Name(w118) -> ("Left"=w120:i16, "Top"=w131:i16)
  n511 = To Word Integer(number=w126) -> (16bit integer=w129:i16)
  n512 = To Word Integer(number=w127) -> (16bit integer=w130:i16)
  n513 = Add(x=w120, y=w123) -> (x+y=w122:i16)
  n514 = Compound Arithmetic op=ADD(w131, w129, w130, i16 12 ("y")) -> (w125:i16)
  n515 = Bundle By Name(cluster=w118, "Right"=w122, "Bottom"=w125) -> (w119:T30)
  n516 = property class="VI"(reference=w117, "Front Panel.PanelBounds"=w119) -> ()  [unwired: 1 in, 2 out]
